vi "AutomatedTransfer_v2.vi"() -> ()   [LabVIEW 2013]
uses:
  controls/Control Configuration.ctl
  controls/Custom Controller Inputs.ctl
  controls/Controller Calcs.ctl
  controls/Observer Calcs.ctl
  controls/Other Calcs.ctl
  controls/UI Data.ctl
  controls/All FPGA Configuration Values.ctl
  controls/FPGA State.ctl
  controls/Raw Values.ctl
  Globals/Global - All UI Loop Stop.vi
  Globals/Global - UI Stream and Variable Connections.vi
  Globals/Global - Configuration Options.vi
  support/User Event - Stop/User Event - Stop.lvlib
  support/Message Queue/Message Queue.lvlib
  <vilib>/Analysis/NI_AALBase.lvlib
panel:
  in  "Switch to Safe State":bool
  in  "Exit":bool
  out "System Status":string="\n8/4/2014 6:26:47 PM: RT Error 91 - Variant To Data in RT Main.vi\n8/4/2014 6:26:32 PM: RT Error 91 - Variant To Data in RT Main.vi\n8/4/2014 6:26:21 PM: RT Error 91 - Variant To Data in RT Main.vi\n8/4/2014 6:26:03 PM: RT Error 91 - Variant To Data in RT Main.vi\n8/4/2014 6:25:47 PM: RT Error 91 - Variant To Data in RT Main.vi\n8/4/2014 6:25:36 PM: RT Error 91 - Variant To Data in RT Main.vi\n6/10/2014 3:19:43 PM: UI Error -1950679035 - Read Variable in AutomatedTransfer_v2.vi\n5/12/2014 3:31:58 PM: UI Error -314220 - Read Single Element from Stream in UI - Read Stream from RT.vi->UI Main.vi\n5/12/2014 3:31:58 PM: UI Error -314220 - Read Single Element from Stream in UI - Read Stream from RT.vi->UI Main.vi\n5/12/2014 3:31:58 PM: UI Error -314220 - Read Single Element from Stream in UI - Read Stream from RT.vi->UI Main.vi\n5/12/2014 3:31:58 PM: UI Error -314220 - Read Single Element from Stream in UI - Read Stream from RT.vi->UI Main.vi\n5/12/2014 3:31:58 PM: UI Error -314220 - Read Single Element from Stream in UI - Read Stream from RT.vi->UI Main.vi\n5/12/2014 3:31:58 PM: UI Error -314220 - Read Single Element from Stream in UI - Read Stream from RT.vi->UI Main.vi\n5/12/2014 3:31:58 PM: UI Error -314220 - Read Single Element from Stream in UI - Read Stream from RT.vi->UI Main.vi\n5/12/2014 3:31:58 PM: UI Error -314220 - Read Single Element from Stream in UI - Read Stream from RT.vi->UI Main.vi\n5/12/2014 3:31:58 PM: UI Error -314220 - Read Single Element from Stream in UI - Read Stream from RT.vi->UI Main.vi\n5/12/2014 3:31:58 PM: UI Error -314220 - Read Single Element from Stream in UI - Read Stream from RT.vi->UI Main.vi\n5/12/2014 3:31:58 PM: UI Error -314220 - Read Single Element from Stream in UI - Read Stream from RT.vi->UI Main.vi\n5/12/2014 3:31:58 PM: UI Error -314220 - Read Single Element from Stream in UI - Read Stream from RT.vi->UI Main.vi\n5/12/2014 3:31:58 PM: UI Error -314220 - Read Single Element from Stream in UI - Read Stream from RT.vi->UI Main.vi\n5/12/2014 3:31:58 PM: UI Error -314220 - Read Single Element from Stream in UI - Read Stream from RT.vi->UI Main.vi\n5/12/2014 3:31:58 PM: UI Error -314220 - Read Single Element from Stream in UI - Read Stream from RT.vi->UI Main.vi\n5/12/2014 3:31:58 PM: UI Error -314220 - Read Single Element from Stream in UI - Read Stream from RT.vi->UI Main.vi\n5/12/2014 3:31:58 PM: UI Error -314220 - Write Single Element to Stream in UI Main.vi\n5/12/2014 3:31:36 PM: UI Error -314004 - Create Network Stream Writer Endpoint in UI - Initiate Connection.vi->UI Main.vi\n5/6/2014 11:02:04 PM: UI Error -314220 - Write Single Element to Stream in UI Main.vi"
  out "Current FPGA Control Mode":u16(ring) items=["Safe State", "Manual", "Control (PID)"]
  in  "Settings Tab":T1(tab)
  out "Stage stop position (mm):":dbl=99.99983984375 format="%#.2g"
  out "Test LED":bool
  out "Roller LED":bool=TRUE
  in  "Test control":bool
  in  "Disable test control":bool
  in  "Stage speed (mm/s):":dbl=21.0 min=0.2 max=21.0
  out "Force results (N)":cluster{dbl[], dbl[]}(graph)
  in  "Save Results":bool
  in  "Stop Test":bool
  in  "Run Test":bool
  in  "Stop dwell time (s):":dbl=2.0 min=0.0
  in  "Start dwell time (s):":dbl=2.0 min=0.0
  in  "Travel distance (mm):":dbl=50.0 min=-150.0 max=150.0 step=0.1
  in  "Contact force (N):":fxp<+/-,20,7>=4.0
  out "Measured contact force (N):":dbl
  out "Stage position (mm):":dbl format="%#.2g"
  out "Fthresh (N):":fxp<+/-,16,8>=2.0 format="%.3g"
  in  "Home position (mm)":dbl=3.5
  in  "Stop roller":bool
  in  "Speed (mm/s):":dbl=2.0 min=0.2 max=5.0
  in  "Contact roller":bool
  in  "Disable roller control":bool
  in  "Roller control":bool
  in  "Home Roller":bool
  in  "Auto tare":bool=TRUE
  out "Position (mm):":dbl
  out "Force (N):":dbl
  out "Max speed (mm/s):":dbl=21.0
  out "Max position (mm):":dbl=151.49760546875
  in  "Position (mm):":dbl=85.0 min=0.0 max=150.0 step=0.1
  in  "Stage speed (mm/s):":dbl=21.0 min=0.2 max=21.0
  out "Stage position (mm):":dbl=99.9996015625 format="%#.2g"
  in  "Go stage":bool
  in  "Stop stage":bool
  in  "Home stage":bool
  out "path":path
  out "Other Calcs":T2
  out "Observer Calcs":T3
  out "Controller Calcs":T4
  in  "Control period (ticks)":u32=40000
  in  "Find tare offset":bool=TRUE
  in  "Channel 3 Setpoint":fxp<+/-,16,5>
  in  "Channel 2 Setpoint":fxp<+/-,16,5>
  in  "Channel 1 Setpoint":fxp<+/-,20,7>=24.0
  in  "Channel 0 Setpoint":fxp<+/-,20,7>=4.0
  in  "Update Control Configuration":bool
  in  "Control Configurations":T5[](array[typedef])=[{"PID Gains"={"proportional gain (Kc)"=55.0, "integral gain (Kc*Ts/Ti)"=0.0, "derivative gain (Kc*Td/Ts)"=0.0}, "Output Range"={"output high"=50.0, "output low"=-50.0}}, {"PID Gains"={"proportional gain (Kc)"=0.0, "integral gain (Kc*Ts/Ti)"=0.0, "derivative gain (Kc*Td/Ts)"=0.0}, "Output Range"={"output high"=10.0, "output low"=-10.0}}, {"PID Gains"={"proportional gain (Kc)"=0.0, "integral gain (Kc*Ts/Ti)"=0.0, "derivative gain (Kc*Td/Ts)"=0.0}, "Output Range"={"output high"=10.0, "output low"=-10.0}}, {"PID Gains"={"proportional gain (Kc)"=0.0, "integral gain (Kc*Ts/Ti)"=0.0, "derivative gain (Kc*Td/Ts)"=0.0}, "Output Range"={"output high"=10.0, "output low"=-10.0}}]
  in  "Run Control":bool
  in  "Stop Control":bool
  in  "Custom Controller Inputs":T6={"Other Controller Gains"={"kvc (N/m)"=1.0, "ymod (-)"=0.0, "Mar (kg)"=0.0, "bp (kg/s)"=0.0, "Foff (N)"=0.16796875, "Fthresh (N)"=2.0}}
  out "Offset (N)":fxp<+/-,16,8>=0.16796875
  in  "Channel 3 Manual Value":fxp<+/-,16,5>
  in  "Channel 2 Manual Value":fxp<+/-,16,5>
  in  "Channel 1 Manual Value":fxp<+/-,16,5>
  in  "Channel 0 Manual Value":fxp<+/-,16,5>
  in  "Run Manual":bool
  in  "Stop Manual":bool
  in  "Retain data":bool
  out "F std":dbl=0.005665196330386121 format="%#_4g"
  out "F avg":dbl=-0.0348828125 format="%#_4g"
  in  "Clear Button":bool
  in  "Pause Button":bool
  in  "Save As Button":bool
  in  "Display frequency (Hz)":dbl=100.0 min=1.0 step=1.0
  out "Inputs (mV or V)":cluster{dbl[], dbl[]}[](graph)
  in  "Number of points":i32=500 min=1 max=999999999
  out "Force (N)":cluster{dbl[], dbl[]}(graph)
  out "V*":cluster{dbl[], dbl[]}(graph)
  out "Roller position (mm)":cluster{dbl[], dbl[]}(graph)
  out "Control loop frequency (Hz)":u32=4294967295
  out "Stage position (mm)":cluster{dbl[], dbl[]}(graph)
  out "Actual Loop Period (ticks)":u32
  out "Largest Contiguous Memory (bytes)":dbl(graph)
  out "CPU Usage (%)":dbl(graph)
  out "Connected?":bool=TRUE
  in  "Connect to Controller":bool
  in  "Controller Address":string="169.254.66.100"
  # "LabVIEW FPGA Control on CompactRIO"
  # "Connection Settings"
  # "Roller panel"
  # "Stage panel"
  # "To do: \n-Update Monitoring Loop Rate by changing Display Rate \n  Note: with 1 ms rate, the program hangs\n-Put 'stage position' in variable references\n-Clean up noise in load cell when V* acts"
  # "Warning: Home cannot be stopped"
  # "Test panel"
  # "Force Command (N)"
  # "Position Command (mm)"
  # "Current Command (Testing)"
  # "Control period and setpoint changes are sent to the target automatically."
  # "Control Configuration changes are sent to the target when you click \"Update Control Configurations\"."
  # "Not used"
  # "Not used"
  # "Not used"
  # "F ="
  # "+/-"
  # "N"
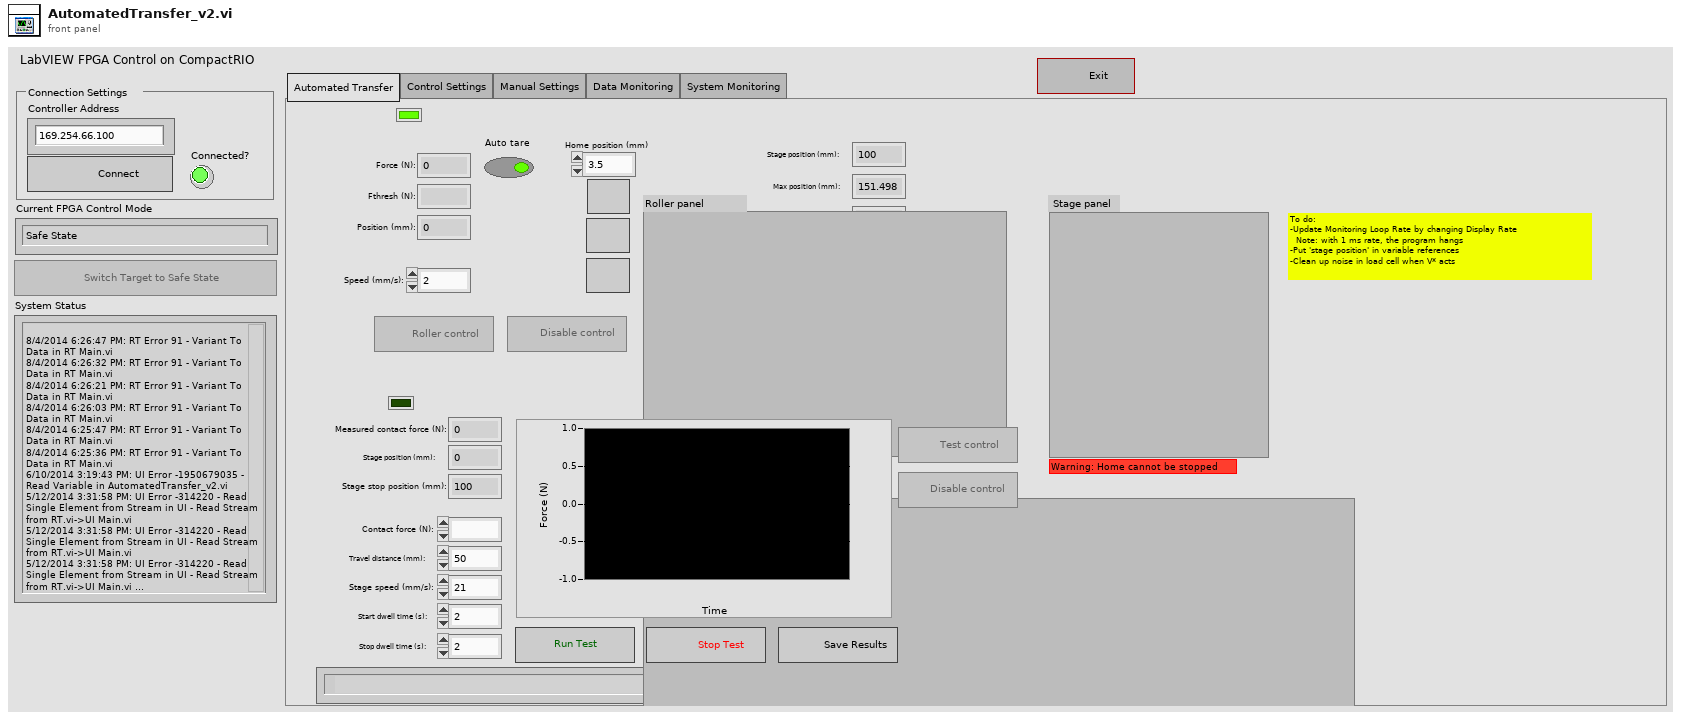
[diagram p1: front panel]
types:
  T1 = enum32{"Automated Transfer", "Control Settings", "Manual Settings", "Data Monitoring", "System Monitoring"}
  T2 = typedef "Other Calcs.ctl" = cluster{"k_1 (1/s)":fxp<+/-,20,7>, "k_2 (1/s)":fxp<+/-,20,7>, "Frr (N/s)":fxp<+/-,20,7>, "xrr (mm/s)":fxp<+/-,20,14>}
  T3 = typedef "Observer Calcs.ctl" = cluster{"bo (kg/s)":fxp<+/-,20,7>, "kso (N/m)":fxp<+/-,20,7>, "kiso (N/m)":fxp<+/-,20,7>}
  T4 = typedef "Controller Calcs.ctl" = cluster{"ba (kg/s)":fxp<+/-,20,7>, "ksa (N/m)":fxp<+/-,20,7>, "kisa (N/m)":fxp<+/-,20,7>, "k_backemf (Vs/m)":fxp<+/-,20,14>}
  T5 = typedef "Control Configuration.ctl" = cluster{"PID Gains":cluster{"proportional gain (Kc)":fxp<+/-,16,8>, "integral gain (Kc*Ts/Ti)":fxp<+/-,16,8>, "derivative gain (Kc*Td/Ts)":fxp<+/-,16,8>}, "Output Range":cluster{"output high":fxp<+/-,16,7>, "output low":fxp<+/-,16,7>}}
  T6 = typedef "Custom Controller Inputs.ctl" = cluster{"Other Controller Gains":cluster{"kvc (N/m)":fxp<+,16,12>, "ymod (-)":fxp<+/-,16,5>, "Mar (kg)":fxp<+/-,16,8>, "bp (kg/s)":fxp<+/-,16,5>, "Foff (N)":fxp<+/-,16,8>, "Fthresh (N)":fxp<+/-,16,5>}}
  T7 = typedef "UI Data.ctl" = cluster{"Switch to Safe State Ref":refnum<vi>, "Run Manual Ref":refnum<vi>, "Stop Manual Ref":refnum<vi>, "Run Control Ref":refnum<vi>, "Stop Control Ref":refnum<vi>, "Update Control Configurations Ref":refnum<vi>, "Ch 0 Setpoint Ref":refnum<vi>, "Ch 1 Setpoint Ref":refnum<vi>, "Ch 2 Setpoint Ref":refnum<vi>, "Ch 3 Setpoint Ref":refnum<vi>, "Ch 0 Manual Ref":refnum<vi>, "Ch 1 Manual Ref":refnum<vi>, "Ch 2 Manual Ref":refnum<vi>, "Ch 3 Manual Ref":refnum<vi>, "Control Configurations Ref":refnum<vi>, "Custom Controller Cluster Ref":refnum<vi>, "Control period (ticks) Ref":refnum<vi>, "Roller control":refnum<vi>, "Disable roller control":refnum<vi>, "Test control":refnum<vi>, "Disable test control":refnum<vi>, "Controller Calcs":refnum<vi>, "Observer Calcs":refnum<vi>, "Other Calcs":refnum<vi>}
  T8 = typedef "Message Queue.lvlib/All Message Queues.ctl" = cluster{"UI":refnum<queue>}
  T9 = enum16{"open", "replace", "create", "open or create", "replace or create", "replace or create with confirmation"}
  T10 = cluster{"Channel 0 Setpoint":fxp<+/-,20,7>, "Channel 1 Setpoint":fxp<+/-,20,7>, "Channel 2 Setpoint":fxp<+/-,16,5>, "Channel 3 Setpoint":fxp<+/-,16,5>}
  T11 = cluster{"Channel 0 Manual Value":fxp<+/-,16,5>, "Channel 1 Manual Value":fxp<+/-,16,5>, "Channel 2 Manual Value":fxp<+/-,16,5>, "Channel 3 Manual Value":fxp<+/-,16,5>}
  T12 = typedef "Variable References.ctl" = cluster{"CPU Usage":refnum<k21>, "Contiguous Memory":refnum<k21>, "Input Values":refnum<k21>, "Output Values":refnum<k21>, "FPGA Mode":refnum<k21>, "Actual Loop Period":refnum<k21>, "Controller Calcs":refnum<k21>, "Observer Calcs":refnum<k21>, "Other Calcs":refnum<k21>}
  T13 = typedef "Raw Values.ctl" = cluster{"Channel 0":fxp<+/-,20,7>, "Channel 1":fxp<+/-,20,7>, "Channel 2":fxp<+/-,20,7>, "Channel 3":fxp<+/-,20,14>}
  T14 = cluster{"Channel 0":dbl, "Channel 1":dbl, "Channel 2":dbl, "Channel 3":dbl}
  T15 = cluster{fxp<+/-,16,5>, "Channel 1 Manual Value":fxp<+/-,16,5>, "Channel 2 Manual Value":fxp<+/-,16,5>, "Channel 3 Manual Value":fxp<+/-,16,5>}
  T16 = cluster{"fixed-point type":fxp<+/-,16,5>, "Channel 1 Manual Value":fxp<+/-,16,5>, "Channel 2 Manual Value":fxp<+/-,16,5>, "Channel 3 Manual Value":fxp<+/-,16,5>}
  T17 = cluster{"Contact force (N): ":fxp<+/-,20,7>, "Channel 1 Setpoint":fxp<+/-,20,7>, "Channel 2 Setpoint":fxp<+/-,16,5>, "Channel 3 Setpoint":fxp<+/-,16,5>}
  T18 = cluster{"Message":string, "Message Data":variant}
  T19 = typedef "All FPGA Configuration Values.ctl" = cluster{"FPGA State":T20, "Manual Values":T13, "Setpoints":T13, "Control Configurations":T5[]}
  T20 = typedef "FPGA State.ctl" = enum16{"Safe State", "Manual", "Control (PID)"}
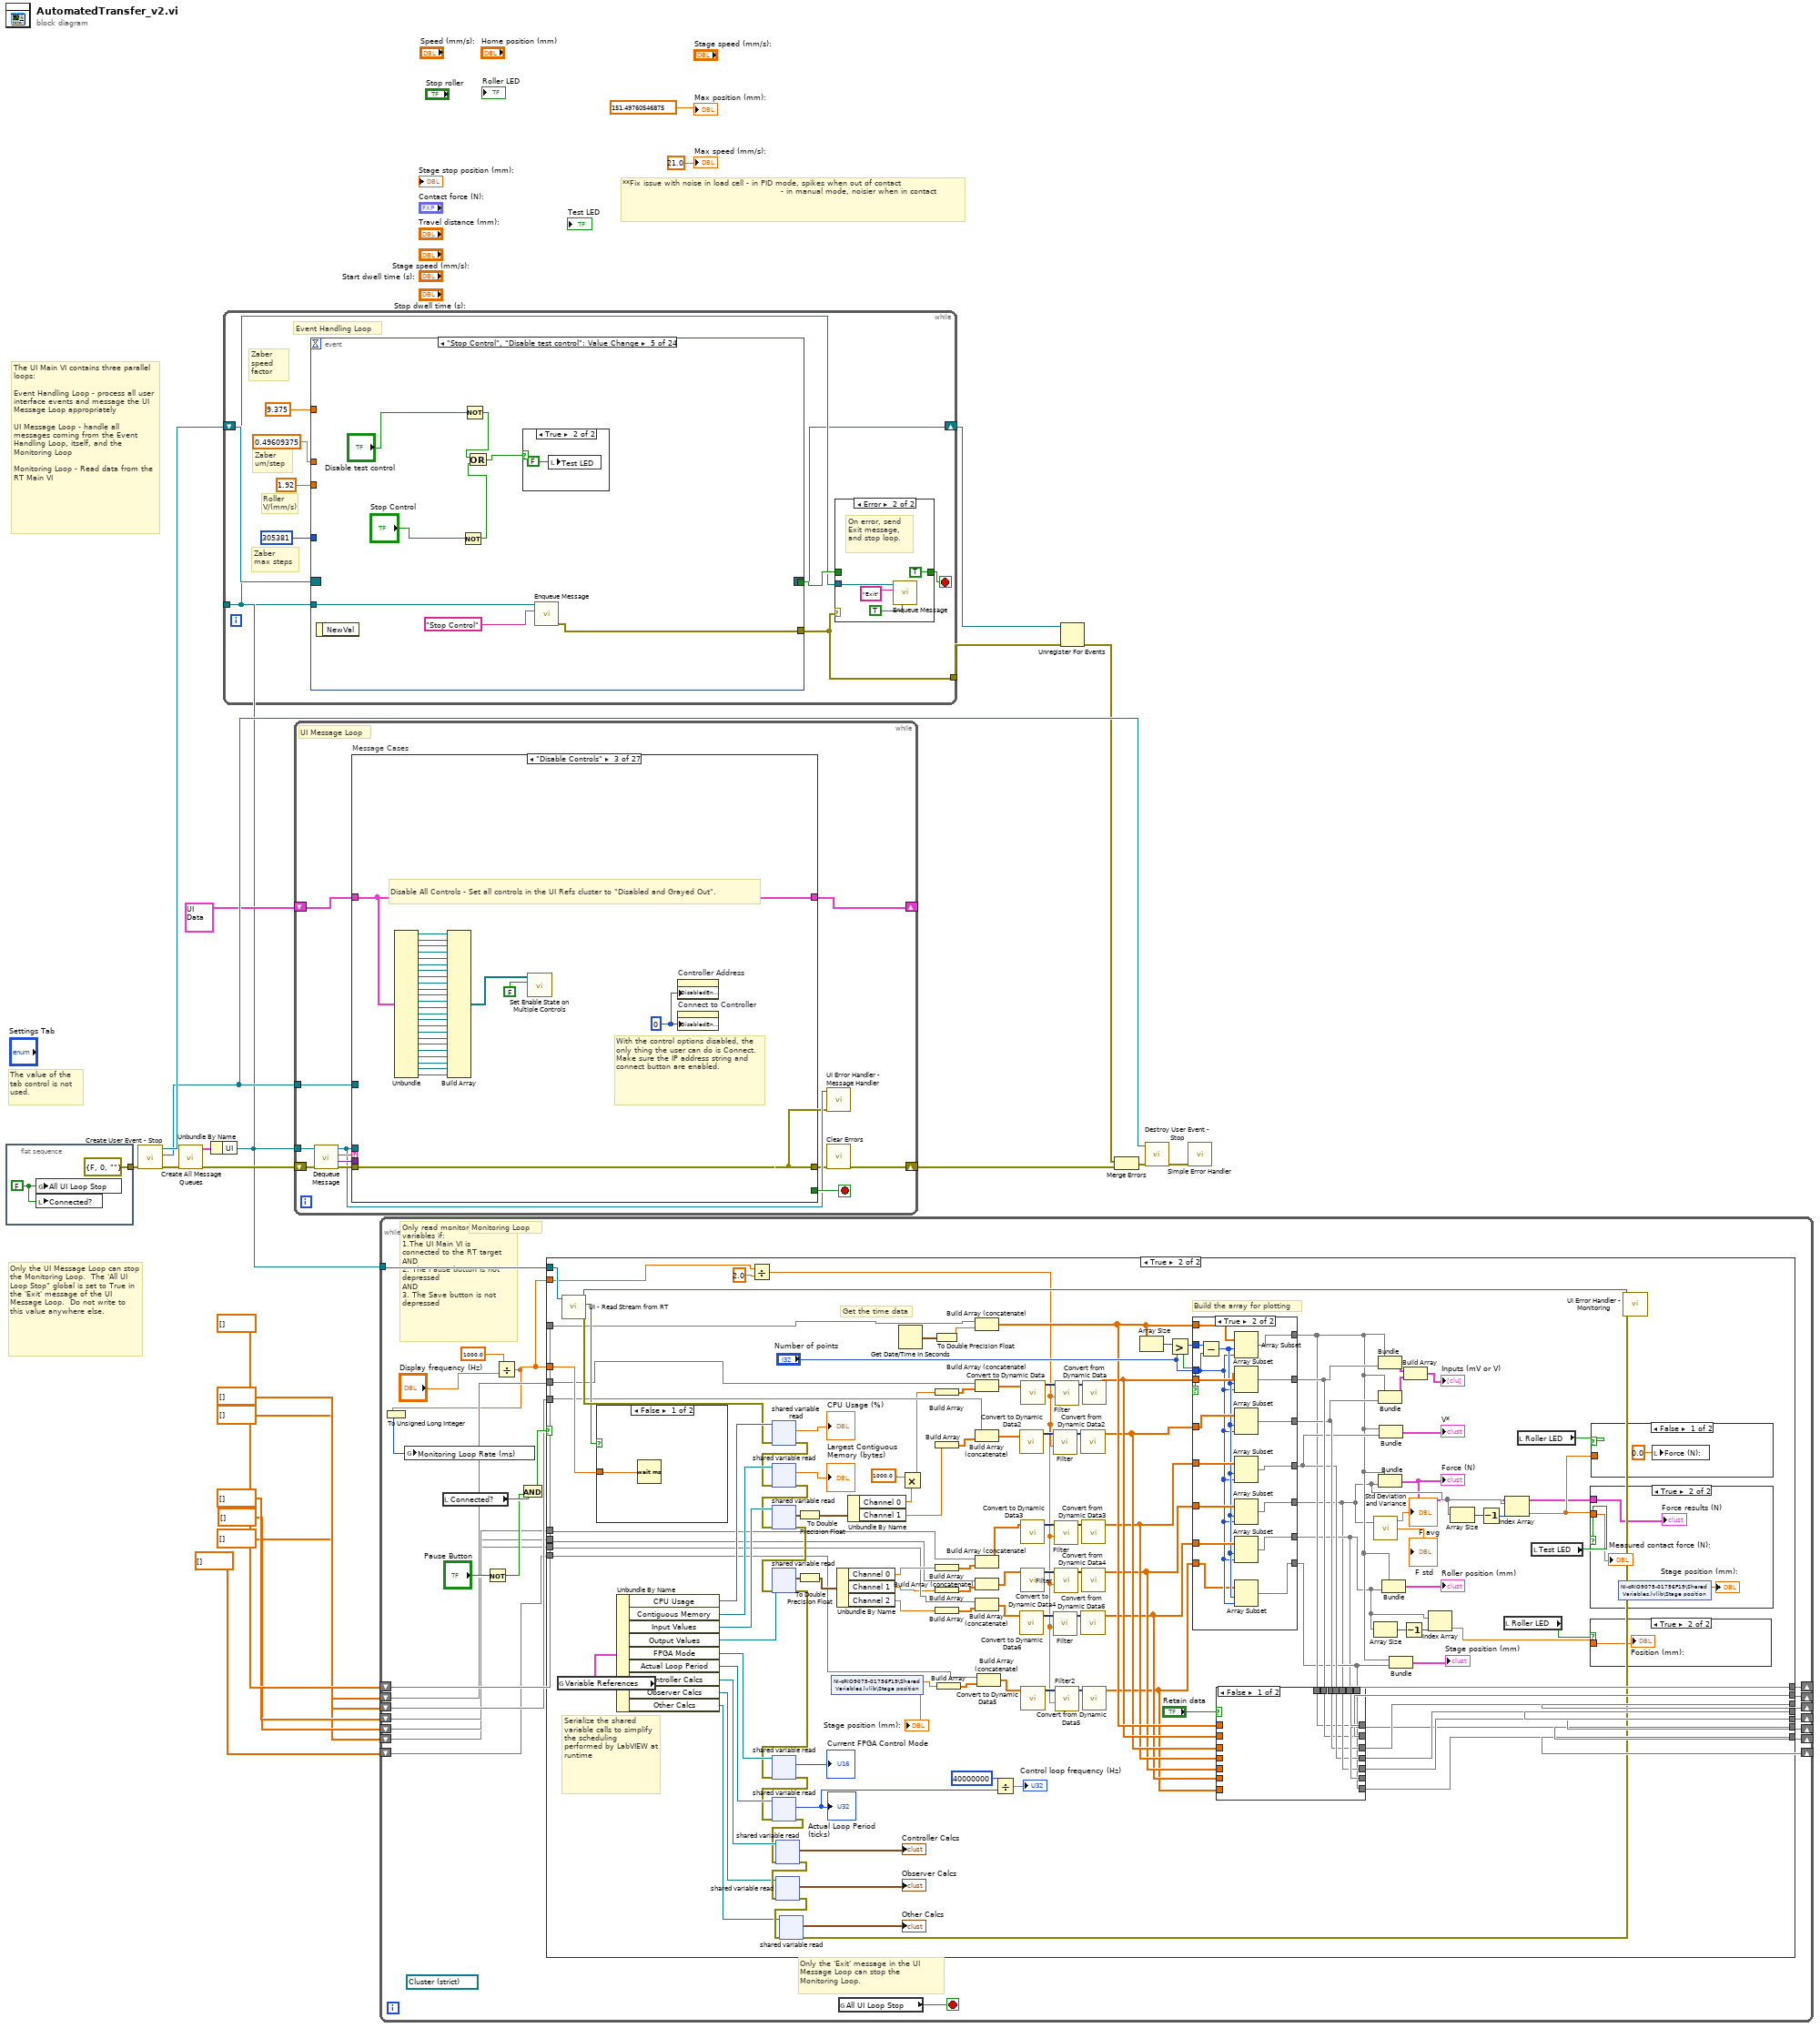
[diagram p0: block diagram]
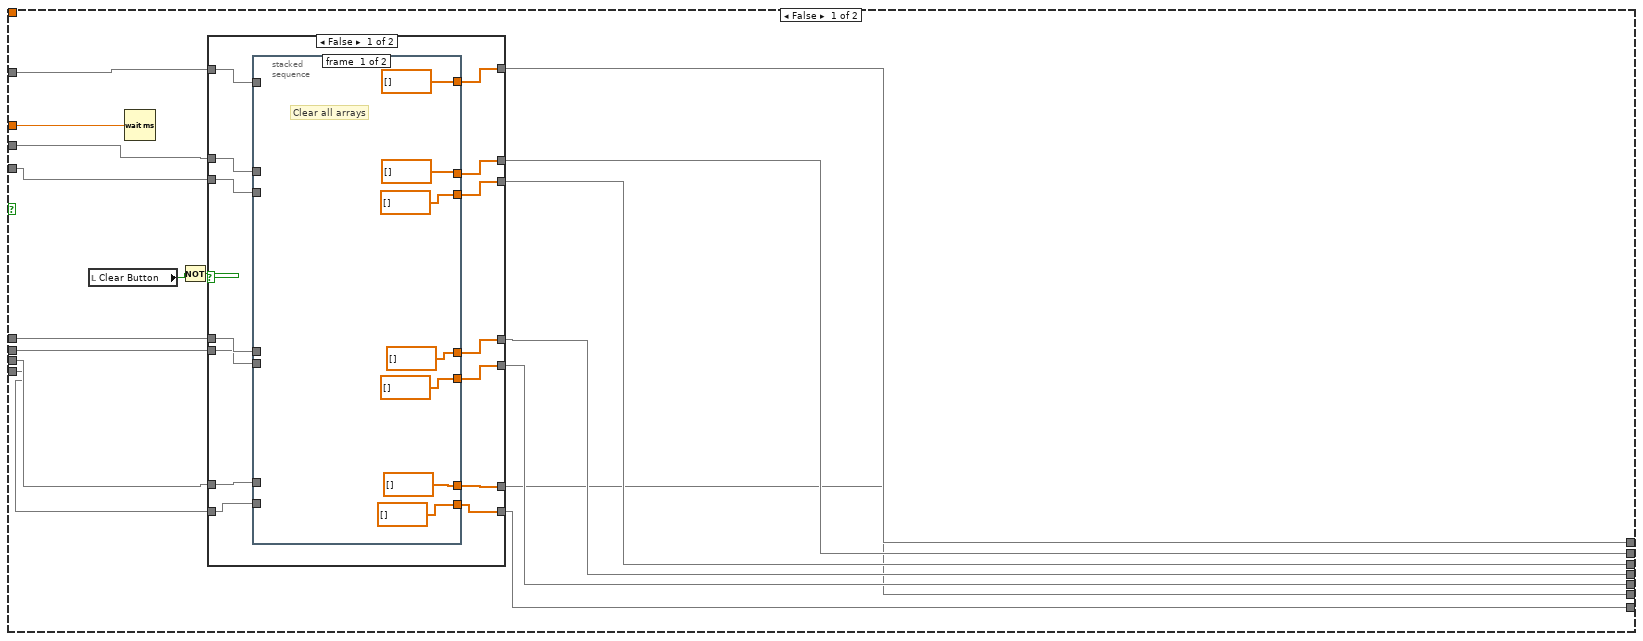
[diagram p2: hidden frame]
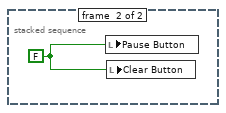
[diagram p3: hidden frame]
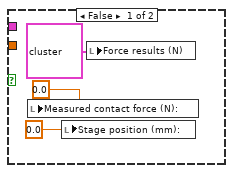
[diagram p5: hidden frame]
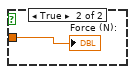
[diagram p6: hidden frame]
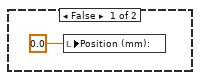
[diagram p7: hidden frame]
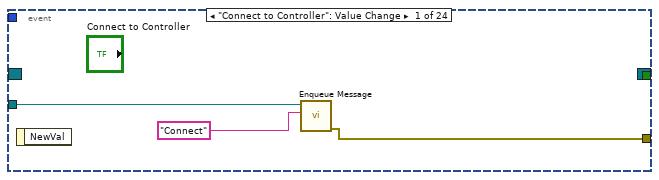
[diagram p12: hidden frame]
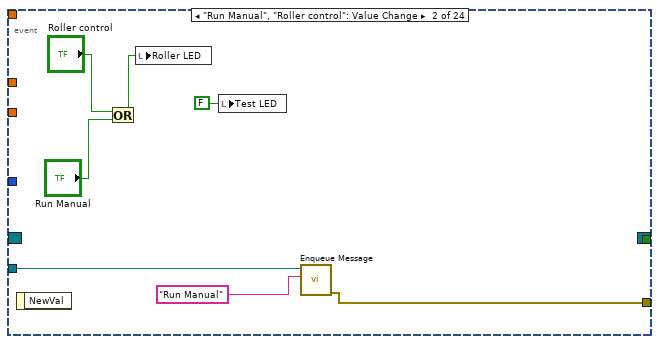
[diagram p13: hidden frame]
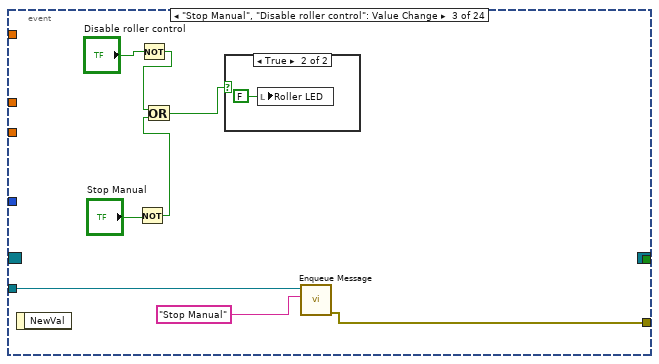
[diagram p14: hidden frame]
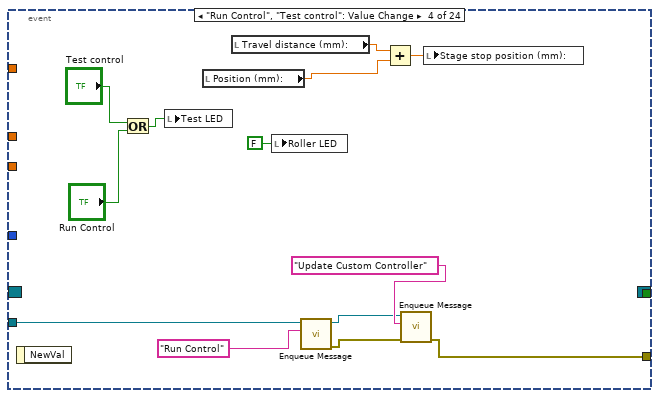
[diagram p16: hidden frame]
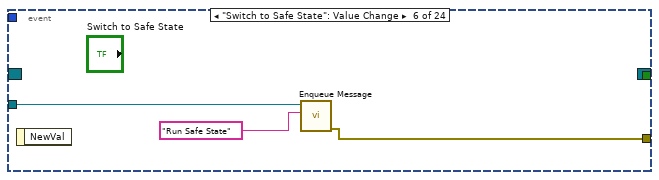
[diagram p18: hidden frame]
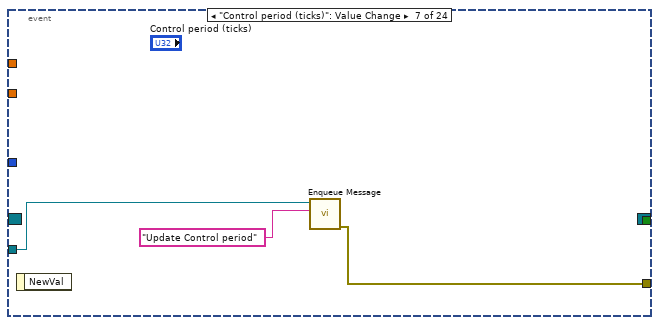
[diagram p19: hidden frame]
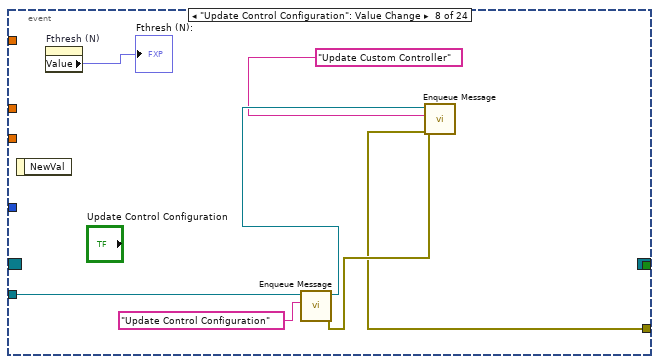
[diagram p20: hidden frame]
diagram:
  # "**Fix issue with noise in load cell - in PID mode, spikes when out of contact\n                                                          - in manual mode, noisier when in contact"
  # "The UI Main VI contains three parallel loops:\n\nEvent Handling Loop - process all user interface events and message the UI Message Loop appropriately\n\nUI Message Loop - handle all messages coming from the Event Handling Loop, itself, and the Monitoring Loop\n\nMonitoring Loop - Read data from the RT Main VI"
  # "The value of the tab control is not used."
  # "Only the UI Message Loop can stop the Monitoring Loop.  The 'All UI Loop Stop\" global is set to True in the 'Exit' message of the UI Message Loop.  Do not write to this value anywhere else."
  n1 = flat-sequence {
    tunnel: [errorcluster {"status"=FALSE, "code"=0, "source"=""} ("error in (no error)")] -> w10
    frame #0 {
      w24 = FALSE
      n2 = global write "Global - All UI Loop Stop.vi" "All UI Loop Stop"(w24) -> ()
      n3 = local write "Connected?"(w24) -> ()
    }
  }
  n4 = call "Create User Event - Stop.vi"("error in (no error)"=w10) -> ("error out"=w18:errorcluster, "User Event - Stop"=w19:refnum<user-event>, "Stop Event Registration Refnum"=w20:refnum<event-registration>)  [unwired: 8 in]
  n5 = call "Create All Message Queues.vi"("error in (no error)"=w18) -> ("error out"=w16:errorcluster, "Message Queues out"=w17:T8)  [unwired: 9 in]
  n6 = Unbundle By Name(w17) -> ("UI"=w11:refnum<queue>)
  n7 = while {
    tunnel: w11 -> [w31]
    tunnel: [w33] -> w22
    shift-right: [w30] -> w14
    shift-left: w20 -> [w32]
    stop <- w34 stop-if-true
    # "Zaber \nmax steps"
    # "Zaber \nspeed factor"
    # "Zaber \num/step"
    # "Roller \nV/(mm/s)"
    # "Event Handling Loop"
    n8 = event shown="[4] \"Stop Control\", \"Disable test control\": Value Change" {
      selector: w32 -> [_ _ _ _ _ _ _ _ _ _ _ _ _ _ _ _ _ _ _ _ _ _ _ _]
      dyn-events: [_ _ _ _ _ _ _ _ _ _ _ _ _ _ _ _ _ _ _ _ _ _ _ _] -> w30
      timeout: _ -> [_ _ _ _ _ _ _ _ _ _ _ _ _ _ _ _ _ _ _ _ _ _ _ _]
      tunnel: [_ _ _ _ _ _ _ _ _ _ _ _ _ _ _ _ _ _ _ _ _ TRUE ("Discard?") _ _] -> w35
      tunnel: w31 -> [w41 w48 w56 w71 w78 w82 w87 w94 w97 w106 w114 w139 w144 w175 w208 w219 w226 w270 w277 _ w296 _ _ _]
      tunnel: [w43 w50 w58 w67 w80 w84 w85 w90 w96 w105 w113 w142 w143 w174 w207 w220 w225 w269 w275 _ _ _ _ _] -> w33
      tunnel: 1.92 -> [_ _ _ _ _ _ _ _ _ _ _ _ _ w173 _ _ _ _ _ _ w295 _ _ _]
      tunnel: 0.49609375 -> [_ _ _ _ _ _ _ _ _ _ _ _ _ _ _ _ w224 _ _ _ w294 _ _ _]
      tunnel: 9.375 -> [_ _ _ _ _ _ _ _ _ _ _ _ _ _ _ _ w223 _ _ _ w293 _ _ _]
      tunnel: 305381 -> [_ _ _ _ _ _ _ _ _ _ _ _ _ _ _ _ w222 _ _ _ w292 _ _ _]
      event "Connect to Controller": Value Change {
        n9 = event-data() -> ()  [unwired: 1 in, 1 out]
        n10 = call "Enqueue Message.vi"("Message"="Connect", "Message Queue"=w41) -> ("error out"=w43:errorcluster)  [unwired: 8 in, 1 out]
      }
      event "Run Manual", "Roller control": Value Change {
        n11 = event-data() -> ()  [unwired: 1 in, 1 out]
        n12 = Or(x="Roller control", y="Run Manual") -> (x .or. y?=w45:bool)
        n13 = local write "Roller LED"(w45) -> ()
        n14 = local write "Test LED"(FALSE ("Test LED")) -> ()
        n15 = call "Enqueue Message.vi"("Message"="Run Manual", "Message Queue"=w48) -> ("error out"=w50:errorcluster)  [unwired: 8 in, 1 out]
      }
      event "Stop Manual", "Disable roller control": Value Change {
        n16 = event-data() -> ()  [unwired: 1 in, 1 out]
        n17 = Not(x="Stop Manual") -> (.not. x?=w53:bool)
        n18 = Not(x="Disable roller control") -> (.not. x?=w52:bool)
        n19 = Or(x=w52, y=w53) -> (x .or. y?=w51:bool)
        n20 = case shown="True" w51 {
          frame False {
          }
          frame True {
            n21 = local write "Roller LED"(FALSE) -> ()
          }
        }
        n22 = call "Enqueue Message.vi"("Message"="Stop Manual", "Message Queue"=w56) -> ("error out"=w58:errorcluster)  [unwired: 8 in, 1 out]
      }
      event "Run Control", "Test control": Value Change {
        n23 = event-data() -> ()  [unwired: 1 in, 1 out]
        n24 = Or(x="Test control", y="Run Control") -> (x .or. y?=w64:bool)
        n25 = local write "Test LED"(w64) -> ()
        n26 = local read "Position (mm):"() -> (w62:dbl)
        n27 = local read "Travel distance (mm):"() -> (w61:dbl)
        n28 = local write "Roller LED"(FALSE ("Roller LED")) -> ()
        n29 = call "Enqueue Message.vi"("Message"="Run Control", "Message Queue"=w71) -> ("error out"=w68:errorcluster, "dup Message Queue"=w69:refnum<queue>)  [unwired: 8 in]
        n30 = Add(x=w61, y=w62) -> (x+y=w60:dbl)
        n31 = call "Enqueue Message.vi"("error in (no error)"=w68, "Message"="Update Custom Controller", "Message Queue"=w69) -> ("error out"=w67:errorcluster)  [unwired: 7 in, 1 out]
        n32 = local write "Stage stop position (mm):"(w60) -> ()
      }
      event "Stop Control", "Disable test control": Value Change {
        n33 = event-data() -> ()  [unwired: 1 in, 1 out]
        n34 = Not(x="Stop Control") -> (.not. x?=w74:bool)
        n35 = Not(x="Disable test control") -> (.not. x?=w75:bool)
        n36 = Or(x=w75, y=w74) -> (x .or. y?=w73:bool)
        n37 = case shown="True" w73 {
          frame False {
          }
          frame True {
            n38 = local write "Test LED"(FALSE) -> ()
          }
        }
        n39 = call "Enqueue Message.vi"("Message"="Stop Control", "Message Queue"=w78) -> ("error out"=w80:errorcluster)  [unwired: 8 in, 1 out]
      }
      event "Switch to Safe State": Value Change {
        n40 = event-data() -> ()  [unwired: 1 in, 1 out]
        n41 = call "Enqueue Message.vi"("Message"="Run Safe State", "Message Queue"=w82) -> ("error out"=w84:errorcluster)  [unwired: 8 in, 1 out]
      }
      event "Control period (ticks)": Value Change {
        n42 = event-data() -> ()  [unwired: 1 in, 1 out]
        n43 = call "Enqueue Message.vi"("Message"="Update Control period", "Message Queue"=w87) -> ("error out"=w85:errorcluster)  [unwired: 8 in, 1 out]
      }
      event "Update Control Configuration": Value Change {
        n44 = event-data() -> ()  [unwired: 1 in, 1 out]
        n45 = property on="Fthresh (N)" class="DigNum (strict)"() -> ("Value"=→"Fthresh (N):":fxp<+/-,16,5>)  [unwired: 2 in, 2 out]
        n46 = call "Enqueue Message.vi"("Message"="Update Control Configuration", "Message Queue"=w94) -> ("error out"=w91:errorcluster, "dup Message Queue"=w92:refnum<queue>)  [unwired: 8 in]
        n47 = call "Enqueue Message.vi"("error in (no error)"=w91, "Message"="Update Custom Controller", "Message Queue"=w92) -> ("error out"=w90:errorcluster)  [unwired: 7 in, 1 out]
      }
      event "Channel 0 Setpoint", "Channel 1 Setpoint", "Channel 2 Setpoint", "Channel 3 Setpoint": Value Change {
        n48 = event-data() -> ()  [unwired: 1 in, 1 out]
        n49 = Bundle("Channel 0 Setpoint"="Channel 0 Setpoint", "Channel 1 Setpoint"="Channel 1 Setpoint", "Channel 2 Setpoint"="Channel 2 Setpoint", "Channel 3 Setpoint"="Channel 3 Setpoint") -> (w95:T10)  [unwired: 1 in]
        n50 = call "Enqueue Message.vi"("Message Data"=w95, "Message"="Update Setpoints", "Message Queue"=w97) -> ("error out"=w96:errorcluster)  [unwired: 7 in, 1 out]
      }
      event "Channel 0 Manual Value", "Channel 1 Manual Value", "Channel 2 Manual Value", "Channel 3 Manual Value": Value Change {
        n51 = event-data() -> ()  [unwired: 1 in, 1 out]
        n52 = Bundle("Channel 0 Manual Value"="Channel 0 Manual Value", "Channel 1 Manual Value"="Channel 1 Manual Value", "Channel 2 Manual Value"="Channel 2 Manual Value", "Channel 3 Manual Value"="Channel 3 Manual Value") -> (w103:T11)  [unwired: 1 in]
        n53 = call "Enqueue Message.vi"("Message Data"=w103, "Message"="Update Manual Values", "Message Queue"=w106) -> ("error out"=w105:errorcluster)  [unwired: 7 in, 1 out]
      }
      event "Find tare offset", "Auto tare": Value Change {
        # "When Auto tare is pressed, the offset force (N) is calculated. This value is automaticaly \ninputted into the Offset weight control of Other Controller Gains."
        n54 = event-data() -> ()  [unwired: 1 in, 1 out]
        n55 = property on="Foff (N)" class="DigNum (strict)"("Value"=fxp<+/-,16,8> 0.0) -> ()  [unwired: 2 in, 2 out]
        n56 = Or(x="Find tare offset", y="Auto tare") -> (x .or. y?=w115:bool)
        n57 = stacked-sequence {
          tunnel: 400 -> [w120 w133 _ _]
          tunnel: w115 -> [w119 _ _ _]
          tunnel: w114 -> [_ _ _ w137]
          tunnel: [_ _ _ w136] -> w113
          frame #0 {
            n58 = case shown="True" w119 {
              tunnel: w120 -> [_ w122]
              frame False {
                n59 = local write "Offset (N)"(0.0 ("Test")) -> ()
              }
              frame True {
                n60 = for {
                  N: w122 -> [_]
                  n61 = global read "Global - UI Stream and Variable Connections.vi" "Variable References"() -> (w126:T12)
                  n62 = Unbundle By Name(w126) -> ("Output Values"=w127:refnum<k21>)
                  n63 = shared-variable-read(w127) -> (w128:T13)  [unwired: 1 in, 3 out]
                  n64 = local read "Offset (N)"() -> (w125:fxp<+/-,16,8>)
                  n65 = To Double Precision Float(number=w128) -> (double precision float=w129:T14)
                  n66 = Unbundle(w129) -> ("Channel 1"=w123:dbl)  [unwired: 3 out]
                  n67 = Add(x=w123, y=w125) -> (x+y=w124:dbl)
                  n68 = local write "Offset (N)"(w124) -> ()
                  n69 = Wait (ms)(milliseconds to wait=u32 5) -> ()  [unwired: 1 out]
                }
              }
            }
          }
          frame #1 {
            n70 = local read "Offset (N)"() -> (w134:fxp<+/-,16,8>)
            n71 = To Double Precision Float(number=w133) -> (double precision float=w132:dbl)
            n72 = Divide(x=w134, y=w132) -> (x/y=w131:dbl)
            n73 = local write "Offset (N)"(w131) -> ()
          }
          frame #2 {
            n74 = local read "Offset (N)"() -> (w135:fxp<+/-,16,8>)
            n75 = property on="Foff (N)" class="DigNum (strict)"("Value"=w135) -> ()  [unwired: 2 in, 2 out]
          }
          frame #3 {
            n76 = call "Enqueue Message.vi"("Message"="Update Custom Controller", "Message Queue"=w137) -> ("error out"=w136:errorcluster)  [unwired: 8 in, 1 out]
          }
        }
        "Offset (N)" <- 0.0 ("Offset weight (N)")
      }
      event "Exit": Value Change {
        w140 = TRUE  # Priority Message
        # "The UI Message Loop handles sending the Exit message to other loops."
        n77 = event-data() -> ()  [unwired: 1 in, 1 out]
        n78 = call "Enqueue Message.vi"("Priority Message? (F)"=w140, "Message"="Exit", "Message Queue"=w139) -> ("error out"=w142:errorcluster)  [unwired: 7 in, 1 out]
      }
      event "Home Roller": Value Change {
        n79 = event-data() -> ()  [unwired: 1 in, 1 out]
        n80 = for {
          N: 3 -> [_]
          tunnel: w144 -> [w147]
          tunnel: [w146] -> w143
          i -> [w148]
          n81 = case shown="2" w148 {
            tunnel: w147 -> [_ w150 _ w170]
            tunnel: [_ w149 _ w169] -> w146
            frame Default {
            }
            frame 0 {
              # "V/(mm/s)"
              n82 = local read "Speed (mm/s):"() -> (w152:dbl)
              n83 = local read "Channel 1 Manual Value"() -> (w157:fxp<+/-,16,5>)
              n84 = local read "Channel 2 Manual Value"() -> (w156:fxp<+/-,16,5>)
              n85 = local read "Channel 3 Manual Value"() -> (w155:fxp<+/-,16,5>)
              n86 = Multiply(x=w152, y=-1.92) -> (x*y=w154:dbl)
              n87 = To Fixed-Point(number=w154) -> (fixed-point=w151:fxp<+/-,16,5>)  [unwired: 1 in]
              n88 = local write "Channel 0 Manual Value"(w151) -> ()
              n89 = Bundle(w151, "Channel 1 Manual Value"=w157, "Channel 2 Manual Value"=w156, "Channel 3 Manual Value"=w155) -> (w158:T15)  [unwired: 1 in]
              n90 = call "Enqueue Message.vi"("Message Data"=w158, "Message"="Home roller", "Message Queue"=w150) -> ("error out"=w149:errorcluster)  [unwired: 7 in, 1 out]
            }
            frame 1 {
              n91 = while {
                stop <- w163 stop-if-true
                n92 = local read "Home position (mm)"() -> (w160:dbl)
                n93 = local read "Position (mm):"() -> (w161:dbl)
                n94 = local read "Stop roller"() -> (w162:bool)
                n95 = Less?(x=w161, y=w160) -> (x < y?=w164:bool)
                n96 = Or(x=w164, y=w162) -> (x .or. y?=w163:bool)
              }
            }
            frame 2 {
              w168 = fxp<+/-,16,5> 0.0 ("fixed-point type")
              n97 = local read "Channel 3 Manual Value"() -> (w165:fxp<+/-,16,5>)
              n98 = local read "Channel 2 Manual Value"() -> (w166:fxp<+/-,16,5>)
              n99 = local read "Channel 1 Manual Value"() -> (w167:fxp<+/-,16,5>)
              n100 = local write "Channel 0 Manual Value"(w168) -> ()
              n101 = Bundle("fixed-point type"=w168, "Channel 1 Manual Value"=w167, "Channel 2 Manual Value"=w166, "Channel 3 Manual Value"=w165) -> (w171:T16)  [unwired: 1 in]
              n102 = call "Enqueue Message.vi"("Message Data"=w171, "Message"="Contact roller", "Message Queue"=w170) -> ("error out"=w169:errorcluster)  [unwired: 7 in, 1 out]
            }
          }
        }
      }
      event "Contact roller": Value Change {
        n103 = event-data() -> ()  [unwired: 1 in, 1 out]
        n104 = for {
          N: 3 -> [_]
          tunnel: w175 -> [w179]
          tunnel: [w178] -> w174
          tunnel: w173 -> [w177]
          i -> [w180]
          n105 = case shown="1" w180 {
            tunnel: w179 -> [_ w183 _ w199]
            tunnel: [_ w182 _ w198] -> w178
            tunnel: w177 -> [_ w181 _ _]
            frame Default {
            }
            frame 0 {
              n106 = local read "Speed (mm/s):"() -> (w188:dbl)
              n107 = local read "Channel 3 Manual Value"() -> (w184:fxp<+/-,16,5>)
              n108 = local read "Channel 1 Manual Value"() -> (w186:fxp<+/-,16,5>)
              n109 = local read "Channel 2 Manual Value"() -> (w185:fxp<+/-,16,5>)
              n110 = Multiply(x=w188, y=w181) -> (x*y=w189:dbl)
              n111 = To Fixed-Point(number=w189) -> (fixed-point=w187:fxp<+/-,16,5>)  [unwired: 1 in]
              n112 = local write "Channel 0 Manual Value"(w187) -> ()
              n113 = Bundle(w187, "Channel 1 Manual Value"=w186, "Channel 2 Manual Value"=w185, "Channel 3 Manual Value"=w184) -> (w190:T15)  [unwired: 1 in]
              n114 = call "Enqueue Message.vi"("Message Data"=w190, "Message"="Contact roller", "Message Queue"=w183) -> ("error out"=w182:errorcluster)  [unwired: 7 in, 1 out]
            }
            frame 1 {
              n115 = while {
                stop <- w194 stop-if-true
                n116 = local read "Fthresh (N):"() -> (w192:fxp<+/-,16,8>)
                n117 = local read "Force (N):"() -> (w197:dbl)
                n118 = local read "Stop roller"() -> (w195:bool)
                n119 = To Double Precision Float(number=w192) -> (double precision float=w193:dbl)
                n120 = Greater?(x=w197, y=w193) -> (0:w196:bool)
                n121 = Or(x=w196, y=w195) -> (x .or. y?=w194:bool)
              }
            }
            frame 2 {
              w200 = fxp<+/-,16,5> 0.0 ("fixed-point type")
              n122 = local read "Channel 1 Manual Value"() -> (w203:fxp<+/-,16,5>)
              n123 = local read "Channel 2 Manual Value"() -> (w202:fxp<+/-,16,5>)
              n124 = local read "Channel 3 Manual Value"() -> (w201:fxp<+/-,16,5>)
              n125 = local write "Channel 0 Manual Value"(w200) -> ()
              n126 = Bundle("fixed-point type"=w200, "Channel 1 Manual Value"=w203, "Channel 2 Manual Value"=w202, "Channel 3 Manual Value"=w201) -> (w204:T16)  [unwired: 1 in]
              n127 = call "Enqueue Message.vi"("Message Data"=w204, "Message"="Contact roller", "Message Queue"=w199) -> ("error out"=w198:errorcluster)  [unwired: 7 in, 1 out]
            }
          }
        }
      }
      event "Stop roller": Value Change {
        n128 = event-data() -> ()  [unwired: 1 in, 1 out]
        n129 = local read "Channel 2 Manual Value"() -> (w210:fxp<+/-,16,5>)
        n130 = local read "Channel 1 Manual Value"() -> (w211:fxp<+/-,16,5>)
        n131 = local read "Channel 3 Manual Value"() -> (w209:fxp<+/-,16,5>)
        n132 = Bundle("fixed-point type"=fxp<+/-,16,5> 0.0, "Channel 1 Manual Value"=w211, "Channel 2 Manual Value"=w210, "Channel 3 Manual Value"=w209) -> (w213:T16)  [unwired: 1 in]
        n133 = call "Enqueue Message.vi"("Message Data"=w213, "Message"="Stop roller", "Message Queue"=w208) -> ("error out"=w207:errorcluster)  [unwired: 7 in, 1 out]
      }
      event "Home stage": Value Change {
        n134 = event-data() -> ()  [unwired: 1 in, 1 out]
        n135 = Bundle(1, 1, 0, 1) -> (w214:cluster{i32, i32, i32, i32})  [unwired: 1 in]
        n136 = call "Enqueue Message.vi"("Message Data"=w214, "Message"="Home stage", "Message Queue"=w219) -> ("error out"=w220:errorcluster)  [unwired: 7 in, 1 out]
      }
      event "Go stage": Value Change {
        n137 = event-data() -> ()  [unwired: 1 in, 1 out]
        n138 = for {
          N: 2 -> [_]
          tunnel: w226 -> [w232]
          tunnel: [w231] -> w225
          tunnel: w224 -> [w230]
          tunnel: w223 -> [w229]
          tunnel: w222 -> [w228]
          i -> [w233]
          n139 = case shown="1" w233 {
            tunnel: w232 -> [_ w248 w261]
            tunnel: [_ w247 w260] -> w231
            tunnel: w230 -> [_ w235 _]
            tunnel: w229 -> [_ w234 _]
            tunnel: w228 -> [_ _ w251]
            frame Default {
            }
            frame 0 {
              n140 = local read "Stage speed (mm/s):"() -> (w241:dbl)
              n141 = Multiply(x=w234, y=w235) -> (x*y=w245:dbl)
              n142 = Divide(x=w245, y=1000.0) -> (x/y=w246:dbl)
              n143 = Divide(x=1.0, y=w246) -> (x/y=w242:dbl)
              n144 = Multiply(x=w241, y=w242) -> (x*y=w240:dbl)
              n145 = To Long Integer(number=w240) -> (32bit integer=w239:i32)
              n146 = Bundle(1, 42, w239, 1) -> (w249:cluster{i32, i32, i32, i32})  [unwired: 1 in]
              n147 = call "Enqueue Message.vi"("Message Data"=w249, "Message"="Update stage speed", "Message Queue"=w248) -> ("error out"=w247:errorcluster)  [unwired: 7 in, 1 out]
            }
            frame 1 {
              n148 = local read "Max position (mm):"() -> (w257:dbl)
              n149 = Divide(x=w251, y=w257) -> (x/y=w258:dbl)
              n150 = Multiply(x="Position (mm):", y=w258) -> (x*y=w259:dbl)
              n151 = To Long Integer(number=w259) -> (32bit integer=w252:i32)
              n152 = Bundle(1, 20, w252, 1) -> (w262:cluster{i32, i32, i32, i32})  [unwired: 1 in]
              n153 = call "Enqueue Message.vi"("Message Data"=w262, "Message"="Go stage", "Message Queue"=w261) -> ("error out"=w260:errorcluster)  [unwired: 7 in, 1 out]
            }
          }
        }
      }
      event "Stop stage", "Stop Test": Value Change {
        n154 = event-data() -> ()  [unwired: 1 in, 1 out]
        n155 = case shown="False" "Stop Test" {
          frame False {
            n156 = local write "Pause Button"(FALSE ("Pause Button")) -> ()
          }
          frame True {
          }
        }
        n157 = Bundle(1, 23, 0, 1) -> (w271:cluster{i32, i32, i32, i32})  [unwired: 1 in]
        n158 = call "Enqueue Message.vi"("Message Data"=w271, "Message"="Stop stage", "Message Queue"=w270) -> ("error out"=w269:errorcluster)  [unwired: 7 in, 1 out]
      }
      event "Contact force (N):": Value Change {
        n159 = event-data() -> ()  [unwired: 1 in, 1 out]
        n160 = local read "Contact force (N):"() -> (w274:fxp<+/-,20,7>)
        n161 = local read "Channel 2 Setpoint"() -> (w279:fxp<+/-,16,5>)
        n162 = local read "Channel 3 Setpoint"() -> (w280:fxp<+/-,16,5>)
        n163 = local read "Channel 1 Setpoint"() -> (w278:fxp<+/-,20,7>)
        n164 = Bundle("Contact force (N):"=w274, "Channel 1 Setpoint"=w278, "Channel 2 Setpoint"=w279, "Channel 3 Setpoint"=w280) -> (w281:T17)  [unwired: 1 in]
        n165 = call "Enqueue Message.vi"("Message Data"=w281, "Message"="Update Setpoints", "Message Queue"=w277) -> ("error out"=w275:errorcluster)  [unwired: 7 in, 1 out]
        n166 = local write "Channel 0 Setpoint"(w274) -> ()
      }
      event "Travel distance (mm):": Value Change {
        # "Keep the inputted travel distance consistent with the range 0-->150 mm"
        n167 = event-data() -> ()  [unwired: 1 in, 1 out]
        n168 = local read "Travel distance (mm):"() -> (w288:dbl)
        n169 = local read "Stage position (mm):"() -> (w289:dbl)
        n170 = Add(x=w289, y=w288) -> (x+y=w282:dbl)
        n171 = Greater?(x=w282, y=0.0) -> (0:w284:bool)
        n172 = Greater Or Equal?(x=150.0, y=w282) -> (x >= y?=w285:bool)
        n173 = And(x=w285, y=w284) -> (x .and. y?=w283:bool)
        n174 = case shown="False" w283 {
          tunnel: w282 -> [w290 w291]
          frame False {
            n175 = local write "Stage stop position (mm):"(w290) -> ()
            n176 = call "Display Message to User"() -> ()  [unwired: 10 in, 2 out]
          }
          frame True {
            n177 = local write "Stage stop position (mm):"(w291) -> ()
          }
        }
      }
      event "Run Test": Value Change {
        n178 = event-data() -> ()  [unwired: 1 in, 1 out]
        n179 = for {
          N: 11 -> [_]
          tunnel: w296 -> [w303]
          tunnel: [w302] -> _
          tunnel: w295 -> [w301]
          tunnel: w294 -> [w300]
          tunnel: w293 -> [w299]
          tunnel: w292 -> [w298]
          i -> [w304]
          n180 = case shown="2" w304 {
            tunnel: w303 -> [_ _ w309 w328 _ _ w344 _ _ _ _ _]
            tunnel: [_ _ w310 w327 _ _ w343 _ _ _ _ _] -> w302
            tunnel: w301 -> [_ _ _ _ _ _ _ _ _ _ _ _]
            tunnel: w300 -> [_ _ w307 _ _ _ _ _ _ _ _ _]
            tunnel: w299 -> [_ _ w308 _ _ _ _ _ _ _ _ _]
            tunnel: w298 -> [_ _ _ _ _ _ w341 _ _ _ _ _]
            frame Default {
            }
            frame 0 {
              w305 = 2
              n181 = property on="Stage speed (mm/s):" class="DigNum (strict)"("DisabledEnum"=w305) -> ()  [unwired: 2 in, 2 out]
              n182 = property on="Position (mm):" class="DigNum (strict)"("DisabledEnum"=w305) -> ()  [unwired: 2 in, 2 out]
              n183 = property on="Contact force (N):" class="DigNum (strict)"("DisabledEnum"=w305) -> ()  [unwired: 2 in, 2 out]
              n184 = property on="Travel distance (mm):" class="DigNum (strict)"("DisabledEnum"=w305) -> ()  [unwired: 2 in, 2 out]
              n185 = property on="Stage speed (mm/s):" class="DigNum (strict)"("DisabledEnum"=w305) -> ()  [unwired: 2 in, 2 out]
              n186 = property on="Start dwell time (s):" class="DigNum (strict)"("DisabledEnum"=w305) -> ()  [unwired: 2 in, 2 out]
              n187 = property on="Stop dwell time (s):" class="DigNum (strict)"("DisabledEnum"=w305) -> ()  [unwired: 2 in, 2 out]
            }
            frame 1 {
              n188 = local read "Stage speed (mm/s):"() -> (w306:dbl)
              n189 = Multiply(x=w308, y=w307) -> (x*y=w314:dbl)
              n190 = Divide(x=w314, y=1000.0) -> (x/y=w313:dbl)
              n191 = Divide(x=1.0, y=w313) -> (x/y=w317:dbl)
              n192 = Multiply(x=w306, y=w317) -> (x*y=w318:dbl)
              n193 = To Long Integer(number=w318) -> (32bit integer=w319:i32)
              n194 = Bundle(1, 42, w319, 1) -> (w312:cluster{i32, i32, i32, i32})  [unwired: 1 in]
              n195 = call "Enqueue Message.vi"("Message Data"=w312, "Message"="Update stage speed", "Message Queue"=w309) -> ("error out"=w310:errorcluster)  [unwired: 7 in, 1 out]
            }
            frame 2 {
              n196 = local read "Channel 3 Setpoint"() -> (w326:fxp<+/-,16,5>)
              n197 = local read "Channel 2 Setpoint"() -> (w325:fxp<+/-,16,5>)
              n198 = local read "Contact force (N):"() -> (w323:fxp<+/-,20,7>)
              n199 = local read "Channel 1 Setpoint"() -> (w324:fxp<+/-,20,7>)
              n200 = Bundle("Contact force (N):"=w323, "Channel 1 Setpoint"=w324, "Channel 2 Setpoint"=w325, "Channel 3 Setpoint"=w326) -> (w329:T17)  [unwired: 1 in]
              n201 = local write "Channel 0 Setpoint"(w323) -> ()
              n202 = call "Enqueue Message.vi"("Message Data"=w329, "Message"="Update Setpoints", "Message Queue"=w328) -> ("error out"=w327:errorcluster)  [unwired: 7 in, 1 out]
            }
            frame 3 {
              n203 = flat-sequence {
                frame #0 {
                  n204 = local write "Number of points"(99999999 ("Number of points")) -> ()
                }
                frame #1 {
                  n205 = local write "Pause Button"(TRUE) -> ()
                  n206 = local write "Clear Button"(TRUE) -> ()
                }
              }
            }
            frame 4 {
              n207 = local read "Start dwell time (s):"() -> (w336:dbl)
              n208 = Multiply(x=w336, y=1000.0) -> (x*y=w335:dbl)
              n209 = Wait (ms)(milliseconds to wait=w335) -> ()  [unwired: 1 out]
            }
            frame 5 {
              n210 = local read "Stage position (mm):"() -> (w337:dbl)
              n211 = local read "Travel distance (mm):"() -> (w339:dbl)
              n212 = local read "Max position (mm):"() -> (w340:dbl)
              n213 = Divide(x=w341, y=w340) -> (x/y=w349:dbl)
              n214 = Add(x=w339, y=w337) -> (x+y=w338:dbl)
              n215 = Multiply(x=w338, y=w349) -> (x*y=w350:dbl)
              n216 = To Long Integer(number=w350) -> (32bit integer=w345:i32)
              n217 = Bundle(1, 20, w345, 1) -> (w342:cluster{i32, i32, i32, i32})  [unwired: 1 in]
              n218 = call "Enqueue Message.vi"("Message Data"=w342, "Message"="Go stage", "Message Queue"=w344) -> ("error out"=w343:errorcluster)  [unwired: 7 in, 1 out]
            }
            frame 6 {
              n219 = while {
                stop <- w369 stop-if-true
                w357 = 100.0 ("y")
                w356 = 100.0 ("x")
                n220 = local read "Stage stop position (mm):"() -> (w361:dbl)
                n221 = shared-variable "NI-cRIO9075-01756F19\\Shared Variables.lvlib\\Stage position"() -> (w358:dbl)  [unwired: 1 in, 1 out]
                n222 = local read "Stop Test"() -> (w365:bool)
                n223 = local read "Test LED"() -> (w367:bool)
                n224 = Multiply(x=w358, y=w356) -> (x*y=w363:dbl)
                n225 = Multiply(x=w361, y=w357) -> (x*y=w362:dbl)
                n226 = Not(x=w367) -> (.not. x?=w364:bool)
                n227 = To Long Integer(number=w363) -> (32bit integer=w360:i32)
                n228 = To Long Integer(number=w362) -> (32bit integer=w355:i32)
                n229 = Divide(x=w355, y=w357) -> (x/y=w354:dbl)
                n230 = Divide(x=w360, y=w356) -> (x/y=w359:dbl)
                n231 = Or(x=w365, y=w364) -> (x .or. y?=w366:bool)
                n232 = To Long Integer(number=w354) -> (32bit integer=w352:i32)
                n233 = To Long Integer(number=w359) -> (32bit integer=w353:i32)
                n234 = Equal?(x=w353, y=w352) -> (x = y?=w368:bool)
                n235 = Or(x=w368, y=w366) -> (x .or. y?=w369:bool)
              }
            }
            frame 7 {
              n236 = local read "Stop Test"() -> (w370:bool)
              n237 = case shown="True" w370 {
                frame False {
                }
                frame True {
                  n238 = local write "Stop dwell time (s):"(0.0 ("Stop dwell time (s):")) -> ()
                }
              }
            }
            frame 8 {
              n239 = local read "Stop dwell time (s):"() -> (w372:dbl)
              n240 = Multiply(x=w372, y=1000.0) -> (x*y=w374:dbl)
              n241 = Wait (ms)(milliseconds to wait=w374) -> ()  [unwired: 1 out]
            }
            frame 9 {
              n242 = local write "Stop Test"(TRUE) -> ()
              n243 = local write "Pause Button"(TRUE) -> ()
            }
            frame 10 {
              w379 = 0
              n244 = local write "Number of points"(500 ("Number of points")) -> ()
              n245 = local write "Travel distance (mm):"(0.0 ("Travel distance (mm):")) -> ()
              n246 = property on="Stage speed (mm/s):" class="DigNum (strict)"("DisabledEnum"=w379) -> ()  [unwired: 2 in, 2 out]
              n247 = property on="Position (mm):" class="DigNum (strict)"("DisabledEnum"=w379) -> ()  [unwired: 2 in, 2 out]
              n248 = property on="Contact force (N):" class="DigNum (strict)"("DisabledEnum"=w379) -> ()  [unwired: 2 in, 2 out]
              n249 = property on="Travel distance (mm):" class="DigNum (strict)"("DisabledEnum"=w379) -> ()  [unwired: 2 in, 2 out]
              n250 = property on="Stage speed (mm/s):" class="DigNum (strict)"("DisabledEnum"=w379) -> ()  [unwired: 2 in, 2 out]
              n251 = property on="Start dwell time (s):" class="DigNum (strict)"("DisabledEnum"=w379) -> ()  [unwired: 2 in, 2 out]
              n252 = property on="Stop dwell time (s):" class="DigNum (strict)"("DisabledEnum"=w379) -> ()  [unwired: 2 in, 2 out]
            }
          }
        }
      }
      event User Event {
        # "The Message Handling Loop processed an \"Exit\" message, which fired this event to stop the Event Handling Loop."
        n253 = event-data() -> ()  [unwired: 1 in, 1 out]
      }
      event "Save As Button", "Save Results": Value Change {
        # "When Save As is pressed, V*, Force, and Position are saved."
        n254 = event-data() -> ()  [unwired: 1 in, 1 out]
        n255 = stacked-sequence {
          frame #0 {
            n256 = call "File Dialog"() -> ("selected path"=w383:path)  [unwired: 12 in, 3 out]
            n257 = local read "Stage position (mm)"() -> (w392:cluster{dbl[], dbl[]})
            n258 = local read "Roller position (mm)"() -> (w391:cluster{dbl[], dbl[]})
            n259 = local read "Force (N)"() -> (w389:cluster{dbl[], dbl[]})
            n260 = local read "V*"() -> (w390:cluster{dbl[], dbl[]})
            n261 = Unbundle(w392) -> (w408:dbl[], w409:dbl[])
            n262 = Unbundle(w389) -> (w394:dbl[])  [unwired: 1 out]
            n263 = Unbundle(w391) -> (w393:dbl[])  [unwired: 1 out]
            n264 = Unbundle(w390) -> (w396:dbl[])  [unwired: 1 out]
            n265 = Array Max & Min(array=w408) -> (min value=w406:dbl)  [unwired: 3 out]
            n266 = Subtract(x=w408, y=w406) -> (x-y=w407:dbl[])
            n267 = Build Array(w407, w409, w394, w393, w396) -> (w412:dbl[][])
            n268 = Build Array("Time (s)" ("element"), "Stage position (mm)" ("element"), "Force (N)" ("element"), "Roller position (mm)" ("element"), "V* (V)" ("element")) -> (w398:string[])
            n269 = Strip Path(path=w383) -> (stripped path=w384:path, name=w387:string)
            n270 = Transpose 2D Array(2D array=w412) -> (transposed array=w410:dbl[][])
            n271 = Concatenate Strings(w387, ".txt" ("name or relative path")) -> (w385:string)
            n272 = Array To Spreadsheet String(array=w398, 3:"%s") -> (spreadsheet string=w401:string)  [unwired: 1 in]
            n273 = local write "Pause Button"(TRUE) -> ()
            n274 = local write "Stop Test"(TRUE) -> ()
            n275 = Build Path(base path=w384, name or relative path=w385) -> (appended path=w381:path)
            "path" <- w381
            n276 = Open/Create/Replace File(file path (use dialog)=w381, operation (0:open)=T9."replace or create with confirmation") -> (refnum out=w382:refnum<file>, error out=w416:errorcluster)  [unwired: 4 in, 1 out]
            n277 = Array To Spreadsheet String(array=w410, 3:"%g" ("format string")) -> (spreadsheet string=w400:string)  [unwired: 1 in]
            n278 = Concatenate Strings(w401, w400) -> (w399:string)
            n279 = Write to Text File(file (use dialog)=w382, text=w399, error in=w416) -> (refnum out=w414:refnum<file>, error out=w415:errorcluster)  [unwired: 2 out]
            n280 = Close File(refnum=w414, error in=w415) -> ()  [unwired: 2 out]
          }
          frame #1 {
            n281 = local read "Save Results"() -> (w418:bool)
            n282 = case shown="True" w418 {
              frame False {
              }
              frame True {
                n283 = Get Date/Time In Seconds() -> (seconds since 1Jan1904=w429:timestamp)
                n284 = local read "Contact force (N):"() -> (w426:fxp<+/-,20,7>)
                n285 = local read "Travel distance (mm):"() -> (w424:dbl)
                n286 = local read "Stage speed (mm/s):"() -> (w423:dbl)
                n287 = local read "path"() -> (w435:path)
                n288 = local read "Start dwell time (s):"() -> (w422:dbl)
                n289 = local read "Stop dwell time (s):"() -> (w421:dbl)
                n290 = Get Date/Time String(seconds (now)=w429) -> (date string=w428:string, time string=w427:string)  [unwired: 2 in]
                n291 = Build Array(w428, w427) -> (w430:string[])
                n292 = Strip Path(path=w435) -> (stripped path=w441:path, name=w440:string)
                n293 = To Double Precision Float(number=w426) -> (double precision float=w425:dbl)
                n294 = Array To Spreadsheet String(array=w430, 3:"%s") -> (spreadsheet string=w431:string)  [unwired: 1 in]
                n295 = Build Array("Setpoint force (N)" ("element"), "Travel distance (mm)" ("element"), "Stage speed (mm/s)" ("element"), "Start dwell time (s)" ("element"), "Stop dwell time (s)" ("element")) -> (w444:string[])
                n296 = Build Array(w425, w424, w423, w422, w421) -> (w420:dbl[])
                n297 = Build Array(w420) -> (w419:dbl[][])
                n298 = Search and Replace String(input string=w440, search string=".txt" ("name or relative path"), replace string="_params.txt" ("name or relative path")) -> (result string=w438:string)  [unwired: 5 in, 3 out]
                n299 = Array To Spreadsheet String(array=w444, 3:"%s") -> (spreadsheet string=w451:string)  [unwired: 1 in]
                n300 = Array To Spreadsheet String(array=w419, 3:"%g" ("format string")) -> (spreadsheet string=w452:string)  [unwired: 1 in]
                n301 = Build Path(base path=w441, name or relative path=w438) -> (appended path=w436:path)
                n302 = Open/Create/Replace File(file path (use dialog)=w436, operation (0:open)=T9."replace or create with confirmation") -> (refnum out=w454:refnum<file>, error out=w443:errorcluster)  [unwired: 4 in, 1 out]
                n303 = Concatenate Strings(w451, w452) -> (w433:string)
                n304 = Concatenate Strings(w431, w433) -> (w432:string)
                n305 = Write to Text File(file (use dialog)=w454, text=w432, error in=w443) -> (refnum out=w456:refnum<file>, error out=w442:errorcluster)  [unwired: 2 out]
                n306 = Close File(refnum=w456, error in=w442) -> ()  [unwired: 2 out]
              }
            }
          }
          frame #2 {
            n307 = local write "Save As Button"(FALSE ("Pause Button")) -> ()
            n308 = local write "Save Results"(FALSE ("Save Results")) -> ()
          }
        }
      }
      event "Clear Button": Value Change {
        # "When the Clear button is pressed, all data are erased."
        n309 = event-data() -> ()  [unwired: 1 in, 1 out]
        n310 = local write "Pause Button"(TRUE) -> ()
      }
    }
    n311 = case shown="Error" w33 {
      tunnel: [w36 TRUE ("Discard?")] -> w34
      tunnel: w35 -> [w36 _]
      tunnel: w31 -> [_ w37]
      frame No Error {
      }
      frame Error {
        # "On error, send Exit message, and stop loop."
        n312 = call "Enqueue Message.vi"("Priority Message? (F)"=TRUE ("Discard?"), "Message"="Exit", "Message Queue"=w37) -> ()  [unwired: 7 in, 2 out]
      }
    }
  }
  n313 = while {
    tunnel: w11 -> [w465]
    tunnel: w19 -> [w470]
    shift-right: [w460] -> w23
    shift-left: w16 -> [w469]
    shift-right: [w463] -> _
    shift-left: T7 {"Switch to Safe State Ref"=refnum, "Run Manual Ref"=refnum, "Stop Manual Ref"=refnum, "Run Control Ref"=refnum, "Stop Control Ref"=refnum, "Update Control Configurations Ref"=refnum, "Ch 0 Setpoint Ref"=refnum, "Ch 1 Setpoint Ref"=refnum, "Ch 2 Setpoint Ref"=refnum, "Ch 3 Setpoint Ref"=refnum, "Ch 0 Manual Ref"=refnum, "Ch 1 Manual Ref"=refnum, "Ch 2 Manual Ref"=refnum, "Ch 3 Manual Ref"=refnum, "Control Configurations Ref"=refnum, "Custom Controller Cluster Ref"=refnum, "Control period (ticks) Ref"=refnum, "Roller control"=refnum, "Disable roller control"=refnum, "Test control"=refnum, "Disable test control"=refnum, "Controller Calcs"=refnum, "Observer Calcs"=refnum, "Other Calcs"=refnum} ("Measurement UI Controls") -> [w464]
    stop <- w471 stop-if-true
    # "UI Message Loop"
    n314 = call "Dequeue Message.vi"("error in (no error)"=w469, "Message Queue"=w465) -> ("error out"=w468:errorcluster, "Message Data"=w466:variant, "Message"=w467:string, "dup Message Queue"=w462:refnum<queue>)  [unwired: 6 in]
    n315 = case "Message Cases" shown="\"Disable Controls\"" w467 {
      selector: w467 -> [_ _ _ _ _ _ _ _ _ w621 _ _ _ _ w687 _ w753 _ _ _ _ _ _ _ _ _ w886]
      tunnel: w462 -> [w473 w488 _ _ w561 _ w579 _ w597 w622 _ _ _ _ _ _ w757 _ _ _ _ _ _ _ w871 _ _]
      tunnel: w468 -> [w475 w506 w535 w545 w566 w577 w581 w586 w617 w624 w642 w653 w664 w675 w688 w712 w767 w788 w798 w810 w820 w834 w846 w857 w876 w881 _]
      tunnel: [w474 w489 w535 w545 w560 w577 w580 w585 w600 w623 w641 w652 w663 w674 w689 w711 w768 w786 w796 w809 w819 w833 w845 w858 w877 w880 w884] -> w461
      tunnel: [_ _ _ _ _ _ _ _ _ _ _ _ _ _ _ _ _ _ _ _ _ _ _ _ TRUE _ _] -> w471
      tunnel: w466 -> [_ _ _ _ _ _ _ _ w615 _ _ _ _ w676 w686 w710 w765 w785 w797 w808 w821 w831 w843 w856 _ _ _]
      tunnel: w470 -> [_ _ _ _ _ _ _ _ _ _ _ _ _ _ _ _ _ _ _ _ _ _ _ _ w875 _ _]
      tunnel: w464 -> [w476 w505 w534 w556 w565 w576 w583 w587 w612 w625 w643 w654 w665 w677 w690 w709 w769 w787 w799 w811 w823 w835 w847 w859 w873 w879 w882]
      tunnel: [w476 w504 w534 w556 w565 w576 w583 w587 w612 w625 w643 w654 w665 w677 w690 w709 w769 w787 w799 w811 w823 w835 w847 w859 w873 w879 w882] -> w463
      frame "Initialize" {
        # "Initialize - Send 'Initialize UI Refs' message to get the UI references bundled and initialized appropriately."
        n316 = call "Enqueue Message.vi"("error in (no error)"=w475, "Message"="Initialize UI Refs", "Message Queue"=w473) -> ("error out"=w474:errorcluster)  [unwired: 7 in, 1 out]
      }
      frame "Initialize UI Refs" {
        # "Send a message to disable them all, since there is no connection at the start."
        # "Initialize UI Refs - Bundle up a cluster of references of all UI elements that are programmatically manipulated."
        n317 = control-ref of="Switch to Safe State"() -> (w503:refnum<vi>)
        n318 = control-ref of="Run Manual"() -> (w502:refnum<vi>)
        n319 = control-ref of="Stop Manual"() -> (w501:refnum<vi>)
        n320 = control-ref of="Run Control"() -> (w500:refnum<vi>)
        n321 = control-ref of="Stop Control"() -> (w499:refnum<vi>)
        n322 = control-ref of="Update Control Configuration"() -> (w498:refnum<vi>)
        n323 = control-ref of="Roller control"() -> (w483:refnum<vi>)
        n324 = control-ref of="Disable roller control"() -> (w482:refnum<vi>)
        n325 = control-ref of="Test control"() -> (w481:refnum<vi>)
        n326 = control-ref of="Disable test control"() -> (w480:refnum<vi>)
        n327 = control-ref of="Observer Calcs"() -> (w478:refnum<vi>)
        n328 = control-ref of="Controller Calcs"() -> (w479:refnum<vi>)
        n329 = control-ref of="Other Calcs"() -> (w477:refnum<vi>)
        n330 = control-ref of="Control period (ticks)"() -> (w484:refnum<vi>)
        n331 = control-ref of="Other Controller Gains"() -> (w485:refnum<vi>)
        n332 = control-ref of="Custom Controller Inputs"() -> ()  [unwired: 1 out]
        n333 = control-ref of="Channel 0 Setpoint"() -> (w497:refnum<vi>)
        n334 = control-ref of="Channel 1 Setpoint"() -> (w496:refnum<vi>)
        n335 = control-ref of="Channel 2 Setpoint"() -> (w495:refnum<vi>)
        n336 = control-ref of="Channel 3 Setpoint"() -> (w494:refnum<vi>)
        n337 = control-ref of="Channel 0 Manual Value"() -> (w493:refnum<vi>)
        n338 = control-ref of="Channel 1 Manual Value"() -> (w492:refnum<vi>)
        n339 = control-ref of="Channel 2 Manual Value"() -> (w491:refnum<vi>)
        n340 = control-ref of="Channel 3 Manual Value"() -> (w490:refnum<vi>)
        n341 = control-ref of="Control Configurations"() -> (w486:refnum<vi>)
        n342 = call "Enqueue Message.vi"("error in (no error)"=w506, "Message"="Disable Controls", "Message Queue"=w488) -> ("error out"=w489:errorcluster)  [unwired: 7 in, 1 out]
        n343 = Bundle By Name(cluster=w505, "Switch to Safe State Ref"=w503, "Run Manual Ref"=w502, "Stop Manual Ref"=w501, "Run Control Ref"=w500, "Stop Control Ref"=w499, "Update Control Configurations Ref"=w498, "Ch 0 Setpoint Ref"=w497, "Ch 1 Setpoint Ref"=w496, "Ch 2 Setpoint Ref"=w495, "Ch 3 Setpoint Ref"=w494, "Ch 0 Manual Ref"=w493, "Ch 1 Manual Ref"=w492, "Ch 2 Manual Ref"=w491, "Ch 3 Manual Ref"=w490, "Control Configurations Ref"=w486, "Custom Controller Cluster Ref"=w485, "Control period (ticks) Ref"=w484, "Roller control"=w483, "Disable roller control"=w482, "Test control"=w481, "Disable test control"=w480, "Controller Calcs"=w479, "Observer Calcs"=w478, "Other Calcs"=w477) -> (w504:T7)
      }
      frame "Disable Controls" {
        w516 = 0
        # "With the control options disabled, the only thing the user can do is Connect. Make sure the IP address string and connect button are enabled."
        # "Disable All Controls - Set all controls in the UI Refs cluster to \"Disabled and Grayed Out\"."
        n344 = Unbundle(w534) -> ("Switch to Safe State Ref"=w533:refnum<vi>, "Run Manual Ref"=w532:refnum<vi>, "Stop Manual Ref"=w531:refnum<vi>, "Run Control Ref"=w530:refnum<vi>, "Stop Control Ref"=w529:refnum<vi>, "Update Control Configurations Ref"=w528:refnum<vi>, "Ch 0 Setpoint Ref"=w527:refnum<vi>, "Ch 1 Setpoint Ref"=w526:refnum<vi>, "Ch 2 Setpoint Ref"=w525:refnum<vi>, "Ch 3 Setpoint Ref"=w524:refnum<vi>, "Ch 0 Manual Ref"=w523:refnum<vi>, "Ch 1 Manual Ref"=w522:refnum<vi>, "Ch 2 Manual Ref"=w521:refnum<vi>, "Ch 3 Manual Ref"=w520:refnum<vi>, "Control Configurations Ref"=w519:refnum<vi>, "Custom Controller Cluster Ref"=w515:refnum<vi>, "Control period (ticks) Ref"=w514:refnum<vi>, "Roller control"=w513:refnum<vi>, "Disable roller control"=w512:refnum<vi>, "Test control"=w511:refnum<vi>, "Disable test control"=w510:refnum<vi>, "Controller Calcs"=w509:refnum<vi>, "Observer Calcs"=w508:refnum<vi>, "Other Calcs"=w507:refnum<vi>)
        n345 = Build Array(w533, w532, w531, w530, w529, w528, w527, w526, w525, w524, w523, w522, w521, w520, w519, w515, w514, w513, w512, w511, w510, w509, w508, w507) -> (w518:refnum<vi>[])
        n346 = call "Set Enable State on Multiple Controls.vi"("Enable?"=FALSE, "Controls"=w518) -> ()  [unwired: 10 in]
        n347 = property on="Controller Address" class="Str"("DisabledEnum"=w516) -> ()  [unwired: 2 in, 2 out]
        n348 = property on="Connect to Controller" class="Bool"("DisabledEnum"=w516) -> ()  [unwired: 2 in, 2 out]
      }
      frame "Enable Configuration Controls" {
        w557 = 2
        # "Once connected, the user shouldn't be able to change the connection settings unless he gets disconnected."
        # "Enable Configuration Controls - After successful connection, ensure appropriate controls are enabled."
        n349 = Unbundle By Name(w556) -> ("Update Control Configurations Ref"=w555:refnum<vi>, "Ch 0 Setpoint Ref"=w554:refnum<vi>, "Ch 1 Setpoint Ref"=w553:refnum<vi>, "Ch 2 Setpoint Ref"=w552:refnum<vi>, "Ch 3 Setpoint Ref"=w551:refnum<vi>, "Ch 0 Manual Ref"=w550:refnum<vi>, "Ch 1 Manual Ref"=w549:refnum<vi>, "Ch 2 Manual Ref"=w548:refnum<vi>, "Ch 3 Manual Ref"=w547:refnum<vi>, "Control Configurations Ref"=w546:refnum<vi>, "Custom Controller Cluster Ref"=w544:refnum<vi>, "Control period (ticks) Ref"=w543:refnum<vi>, "Roller control"=w542:refnum<vi>, "Disable roller control"=w541:refnum<vi>, "Test control"=w540:refnum<vi>, "Disable test control"=w539:refnum<vi>, "Controller Calcs"=w538:refnum<vi>, "Observer Calcs"=w537:refnum<vi>, "Other Calcs"=w536:refnum<vi>)
        n350 = Build Array(w555, w554, w553, w552, w551, w550, w549, w548, w547, w546, w544, w543, w542, w541, w540, w539, w538, w537, w536) -> (w559:refnum<vi>[])
        n351 = call "Set Enable State on Multiple Controls.vi"("Enable?"=TRUE, "Controls"=w559) -> ()  [unwired: 10 in]
        n352 = property on="Controller Address" class="Str"("DisabledEnum"=w557) -> ()  [unwired: 2 in, 2 out]
        n353 = property on="Connect to Controller" class="Bool"("DisabledEnum"=w557) -> ()  [unwired: 2 in, 2 out]
      }
      frame "Connect" {
        # "Connect - Attempt to connect to both streams, and the variables, on the RT target."
        n354 = call "UI - Initiate Connection.vi"("error in (no error)"=w566, "Controller Address"="Controller Address", "Message Queue"=w561) -> ("error out"=w563:errorcluster, "Connected?"=w562:bool)  [unwired: 7 in]
        "Connected?" <- w562
        n355 = case shown="True" w562 {
          tunnel: w563 -> [w567 w571]
          tunnel: w561 -> [_ w570]
          tunnel: [w567 w569] -> w560
          frame False {
          }
          frame True {
            n356 = call "Enqueue Message.vi"("error in (no error)"=w571, "Message"="Enable Configuration Controls", "Message Queue"=w570) -> ("error out"=w569:errorcluster)  [unwired: 7 in, 1 out]
          }
        }
      }
      frame "Close Connections" {
        # "Close Connections - Close the connections shared with the Monitoring Loop."
        n357 = global read "Global - UI Stream and Variable Connections.vi" "UI Command Stream"() -> (w575:refnum<k21>)
        n358 = global read "Global - UI Stream and Variable Connections.vi" "RT Message Stream"() -> (w574:refnum<k21>)
        n359 = global read "Global - UI Stream and Variable Connections.vi" "Variable References"() -> (w573:T12)
        n360 = local write "Connected?"(FALSE ("Connected?")) -> ()
        n361 = Destroy Stream Endpoint(11:w575) -> ()  [unwired: 1 in, 1 out]
        n362 = Destroy Stream Endpoint(11:w574) -> ()  [unwired: 1 in, 1 out]
        n363 = call "Close Variable Connections.vi"("Variable References"=w573) -> ()  [unwired: 11 in]
      }
      frame "Disconnect UI" {
        # "Disconnect UI - Something has gone wrong with the connection. Reinitialize the UI to its disconnected state."
        n364 = local write "Connected?"(FALSE ("Connected?")) -> ()
        n365 = call "Enqueue Message.vi"("error in (no error)"=w581, "Message"="Disable Controls", "Message Queue"=w579) -> ("error out"=w580:errorcluster)  [unwired: 7 in, 1 out]
      }
      frame "Get Settings from FPGA" {
        # "Get Settings from FPGA - Send a command to the RT to retrieve all current FPGA Main VI parameter values and send them back to the UI."
        n366 = local read "Connected?"() -> (w584:bool)
        n367 = case shown="True" w584 {
          tunnel: w586 -> [w588 w592]
          tunnel: [w588 w591] -> w585
          frame False {
            # "Don't bother trying to send a message to the RT system if UI Main VI isn't even connected"
          }
          frame True {
            n368 = global read "Global - UI Stream and Variable Connections.vi" "UI Command Stream"() -> (w589:refnum<k21>)
            n369 = shared-variable-write(w589, w592, T18 {"Message"="Send FPGA Configuration to UI", "Message Data"=variant} ("data in")) -> (w591:errorcluster)  [unwired: 1 in, 2 out]
          }
        }
      }
      frame "Initial UI Values" {
        # "Initial UI Values - These are the current values of the FPGA Main VI's R/W controls. They are used to initialize the panel of UI Main VI upon successful connection to the RT target."
        # "Set values of all manual and setpoint controls via reference."
        n370 = Variant To Data(error in=w617, type=T19 {"FPGA State"=enum."Safe State", "Manual Values"={"Channel 0"=0.0, "Channel 1"=0.0, "Channel 2"=0.0, "Channel 3"=0.0}, "Setpoints"={"Channel 0"=0.0, "Channel 1"=0.0, "Channel 2"=0.0, "Channel 3"=0.0}, "Control Configurations"=[]} ("All FPGA Configuration Values"), Variant=w615) -> (data=w613:T19, error out=w616:errorcluster)
        n371 = Unbundle By Name(w612) -> ("Ch 0 Setpoint Ref"=w611:refnum<vi>, "Ch 1 Setpoint Ref"=w610:refnum<vi>, "Ch 2 Setpoint Ref"=w609:refnum<vi>, "Ch 3 Setpoint Ref"=w608:refnum<vi>, "Ch 0 Manual Ref"=w607:refnum<vi>, "Ch 1 Manual Ref"=w606:refnum<vi>, "Ch 2 Manual Ref"=w605:refnum<vi>, "Ch 3 Manual Ref"=w604:refnum<vi>)
        n372 = Unbundle By Name(w613) -> ("Setpoints"=w595:T13, "Manual Values"=w593:T13, "Control Configurations"=w601:T5[], "FPGA State"=w598:T20)
        n373 = Build Array(w611, w610, w609, w608, w607, w606, w605, w604) -> (w603:refnum<vi>[])
        n374 = To Variant(anything=w593) -> (Variant=w594:variant)
        n375 = To Variant(anything=w595) -> (Variant=w596:variant)
        n376 = local write "Current FPGA Control Mode"(w598) -> ()
        n377 = Build Array(w596, w594) -> (w602:variant[])
        n378 = local write "Control Configurations"(w601) -> ()
        n379 = for {
          tunnel: w603 -> [w619] mode=indexing
          tunnel: w602 -> [w618] mode=indexing
          n380 = property class="DigNum"(reference=w619, "Value"=w618) -> ()  [unwired: 1 in, 2 out]
        }
        n381 = call "Enqueue Message.vi"("error in (no error)"=w616, "Message Data"=w598, "Message"="Update Display Mode", "Message Queue"=w597) -> ("error out"=w600:errorcluster)  [unwired: 6 in, 1 out]
      }
      frame "Run Control", "Run Manual", "Run Safe State", "Stop Control", "Stop Manual" {
        # "Run/Stop buttons - Send a command to switch the FPGA into the appropriate state. Send a message to update this UI to reflect the new state."
        n382 = local read "Connected?"() -> (w620:bool)
        n383 = case shown="True" w620 {
          tunnel: w624 -> [w626 w636]
          tunnel: [w626 w632] -> w623
          tunnel: w622 -> [_ w631]
          tunnel: w621 -> [_ w630]
          frame False {
            # "Don't bother trying to send a message to the RT system if UI Main VI isn't even connected"
          }
          frame True {
            # "Run Manual and Run Control switch into their respective states. Anything else switches to Safe State."
            n384 = case shown="\"Run Control\"" w630 {
              tunnel: [FPGA_State."Safe State" ("FPGA State") FPGA_State."Control (PID)" ("FPGA State") FPGA_State."Manual" ("FPGA State")] -> w627
              frame "Safe State", "Stop Control", "Stop Manual", Default {
              }
              frame "Run Control" {
              }
              frame "Run Manual" {
              }
            }
            n385 = global read "Global - UI Stream and Variable Connections.vi" "UI Command Stream"() -> (w628:refnum<k21>)
            n386 = Bundle("Update FPGA State", "FPGA State"=w627) -> (w633:cluster{string, "FPGA State":T20})  [unwired: 1 in]
            n387 = shared-variable-write(w628, w636, w633) -> (w635:errorcluster)  [unwired: 1 in, 2 out]
            n388 = call "Enqueue Message.vi"("error in (no error)"=w635, "Message Data"=w627, "Message"="Update Display Mode", "Message Queue"=w631) -> ("error out"=w632:errorcluster)  [unwired: 6 in, 1 out]
          }
        }
      }
      frame "Update Control period" {
        n389 = local read "Connected?"() -> (w640:bool)
        n390 = case shown="True" w640 {
          tunnel: w642 -> [w644 w650]
          tunnel: [w644 w649] -> w641
          frame False {
            # "Don't bother trying to send a message to the RT system if UI Main VI isn't even connected"
          }
          frame True {
            n391 = global read "Global - UI Stream and Variable Connections.vi" "UI Command Stream"() -> (w646:refnum<k21>)
            n392 = local read "Control period (ticks)"() -> (w645:u32)
            n393 = Bundle("Update Control period", "Control period (ticks)"=w645) -> (w647:cluster{string, "Control period (ticks)":u32})  [unwired: 1 in]
            n394 = shared-variable-write(w646, w650, w647) -> (w649:errorcluster)  [unwired: 1 in, 2 out]
          }
        }
      }
      frame "Update Control Configuration" {
        # "Update Control Configuration - Send all control configurations to RT to be sent down to the FPGA."
        n395 = local read "Connected?"() -> (w651:bool)
        n396 = case shown="True" w651 {
          tunnel: w653 -> [w655 w661]
          tunnel: [w655 w660] -> w652
          frame False {
            # "Don't bother trying to send a message to the RT system if UI Main VI isn't even connected"
          }
          frame True {
            n397 = global read "Global - UI Stream and Variable Connections.vi" "UI Command Stream"() -> (w656:refnum<k21>)
            n398 = Bundle("Update Control Configurations", "Control Configurations"="Control Configurations") -> (w658:cluster{string, "Control Configurations":T5[]})  [unwired: 1 in]
            n399 = shared-variable-write(w656, w661, w658) -> (w660:errorcluster)  [unwired: 1 in, 2 out]
          }
        }
      }
      frame "Update Custom Controller" {
        # "Update Control Configuration - Send all control configurations to RT to be sent down to the FPGA."
        n400 = local read "Connected?"() -> (w662:bool)
        n401 = case shown="True" w662 {
          tunnel: w664 -> [w666 w672]
          tunnel: [w666 w671] -> w663
          frame False {
            # "Don't bother trying to send a message to the RT system if UI Main VI isn't even connected"
          }
          frame True {
            n402 = global read "Global - UI Stream and Variable Connections.vi" "UI Command Stream"() -> (w668:refnum<k21>)
            n403 = Bundle("Update Custom Controller", "Custom Controller Inputs"="Custom Controller Inputs") -> (w669:cluster{string, "Custom Controller Inputs":T6})  [unwired: 1 in]
            n404 = shared-variable-write(w668, w672, w669) -> (w671:errorcluster)  [unwired: 1 in, 2 out]
          }
        }
      }
      frame "Update stage speed" {
        n405 = local read "Connected?"() -> (w673:bool)
        n406 = case shown="True" w673 {
          tunnel: w675 -> [w678 w684]
          tunnel: [w678 w683] -> w674
          tunnel: w676 -> [_ w679]
          frame False {
            # "Don't bother trying to send a message to the RT system if UI Main VI isn't even connected"
          }
          frame True {
            n407 = global read "Global - UI Stream and Variable Connections.vi" "UI Command Stream"() -> (w680:refnum<k21>)
            n408 = Bundle("Update stage speed", "Message Data"=w679) -> (w681:cluster{string, "Message Data":variant})  [unwired: 1 in]
            n409 = shared-variable-write(w680, w684, w681) -> (w683:errorcluster)  [unwired: 1 in, 2 out]
          }
        }
      }
      frame "Update Manual Values", "Update Setpoints" {
        # "Update Manual Values/Setpoints - Send all manual values/setpoints to RT to be sent down to the FPGA."
        n410 = local read "Connected?"() -> (w685:bool)
        n411 = case shown="True" w685 {
          tunnel: [w691 w697] -> w689
          tunnel: w688 -> [w691 w695]
          tunnel: w687 -> [_ w694]
          tunnel: w686 -> [_ w693]
          frame False {
            # "Don't bother trying to send a message to the RT system if UI Main VI isn't even connected"
          }
          frame True {
            n412 = global read "Global - UI Stream and Variable Connections.vi" "UI Command Stream"() -> (w692:refnum<k21>)
            n413 = Bundle(w694, "Message Data"=w693) -> (w696:cluster{string, "Message Data":variant})  [unwired: 1 in]
            n414 = shared-variable-write(w692, w695, w696) -> (w697:errorcluster)  [unwired: 1 in, 2 out]
          }
        }
      }
      frame "Update Display Mode" {
        # "Update Display Mode - Enable/Disable Controls appropriately for the new display mode."
        n415 = Variant To Data(error in=w712, type=FPGA_State."Safe State" ("FPGA State"), Variant=w710) -> (data=w708:T20, error out=w711:errorcluster)
        n416 = Unbundle By Name(w709) -> ("Switch to Safe State Ref"=w707:refnum<vi>, "Run Manual Ref"=w706:refnum<vi>, "Stop Manual Ref"=w705:refnum<vi>, "Run Control Ref"=w704:refnum<vi>, "Stop Control Ref"=w703:refnum<vi>, "Roller control"=w701:refnum<vi>, "Disable roller control"=w700:refnum<vi>, "Test control"=w699:refnum<vi>, "Disable test control"=w698:refnum<vi>)
        n417 = case shown="\"Safe State\"" w708 {
          tunnel: w707 -> [w721 w734 w745]
          tunnel: w706 -> [w717 w733 w747]
          tunnel: w705 -> [w720 w732 w744]
          tunnel: w704 -> [w719 w730 w746]
          tunnel: w703 -> [w718 w731 w743]
          tunnel: w701 -> [w715 w729 w742]
          tunnel: w700 -> [w714 w728 w741]
          tunnel: w699 -> [w716 w727 w740]
          tunnel: w698 -> [w713 w726 w739]
          frame "Control (PID)" {
            n418 = Build Array "Controls to Enable"(w721, w718, w717, w715, w713) -> (w725:refnum<vi>[])
            n419 = Build Array "Controls to Disable"(w720, w719, w716, w714) -> (w723:refnum<vi>[])
            n420 = call "Set Enable State on Multiple Controls.vi"("Enable?"=FALSE, "Controls"=w723) -> ()  [unwired: 10 in]
            n421 = call "Set Enable State on Multiple Controls.vi"("Enable?"=TRUE, "Controls"=w725) -> ()  [unwired: 10 in]
          }
          frame "Manual" {
            n422 = Build Array "Controls to Enable"(w734, w732, w730, w728, w727) -> (w738:refnum<vi>[])
            n423 = Build Array "Controls to Disable"(w733, w731, w729, w726) -> (w736:refnum<vi>[])
            n424 = call "Set Enable State on Multiple Controls.vi"("Enable?"=FALSE, "Controls"=w736) -> ()  [unwired: 10 in]
            n425 = call "Set Enable State on Multiple Controls.vi"("Enable?"=TRUE, "Controls"=w738) -> ()  [unwired: 10 in]
          }
          frame "Safe State" {
            # "This frame runs when FPGA is in Safe State. Only enable the two run buttons."
            n426 = Build Array "Controls to Enable"(w747, w746, w742, w740) -> (w751:refnum<vi>[])
            n427 = Build Array "Controls to Disable"(w745, w744, w743, w741, w739) -> (w749:refnum<vi>[])
            n428 = call "Set Enable State on Multiple Controls.vi"("Enable?"=FALSE, "Controls"=w749) -> ()  [unwired: 10 in]
            n429 = call "Set Enable State on Multiple Controls.vi"("Enable?"=TRUE, "Controls"=w751) -> ()  [unwired: 10 in]
          }
        }
      }
      frame "Critical Error", "Log-Only Error", "Non-Critical Error", "RT Error" {
        # "Error - Display message in status indicator on panel.  If it's a critical error, shut down this VI with an 'Exit' message."
        n430 = case shown="Default" w753 {
          selector: w753 -> [_ w771]
          tunnel: ["UI Error" w771] -> w752
          frame Default {
          }
          frame "RT Error" {
          }
        }
        n431 = Variant To Data(error in=w767, type=errorcluster {"status"=FALSE, "code"=0, "source"=""} ("error constant"), Variant=w765) -> (data=w760:errorcluster, error out=w766:errorcluster)
        n432 = Unbundle By Name(w760) -> ("code"=w759:i32, "source"=w763:string)
        n433 = Format Date/Time String() -> (date/time string=w762:string)  [unwired: 3 in]
        n434 = Format Into String(format string="\n%s: %s %d - %s", w762, w752, w759, w763) -> (resulting string=w754:string)  [unwired: 2 in, 1 out]
        n435 = call "Enqueue Message.vi"("error in (no error)"=w766, "Message Data"=w754, "Message"="Update System Status", "Message Queue"=w757) -> ("error out"=w758:errorcluster, "dup Message Queue"=w756:refnum<queue>)  [unwired: 6 in]
        n436 = case shown="Default" w753 {
          tunnel: w758 -> [w772 w776]
          tunnel: w756 -> [_ w774]
          tunnel: [w772 w775] -> w768
          frame Default {
          }
          frame "Critical Error" {
            n437 = call "Enqueue Message.vi"("error in (no error)"=w776, "Message"="Exit", "Message Queue"=w774) -> ("error out"=w775:errorcluster)  [unwired: 7 in, 1 out]
          }
        }
      }
      frame "Update System Status" {
        # "Code Recommended - The code below ensures that the System Status string value does not become too large.  It uses the same maximum size as the RT error log to determine whether or not to remove the last half of the log string. Change this logic if you wish to maintain more/less of the information in the System Status string."
        # "Update System Status - Add a new string to the beginning of the System Status string on the UI."
        n438 = Variant To Data(error in=w788, type="", Variant=w785) -> (data=w782:string, error out=w786:errorcluster)
        n439 = local read "System Status"() -> (w780:string)
        n440 = global read "Global - Configuration Options.vi" "Error Log Max Size (bytes)"() -> (w778:i64)
        n441 = String Length(string=w780) -> (length=w781:i32)
        n442 = Greater?(x=w781, y=w778) -> (0:w779:bool)
        n443 = case shown="True" w779 {
          tunnel: w780 -> [w789 w793]
          tunnel: w778 -> [_ w792]
          tunnel: [w789 w794] -> w777
          frame False {
          }
          frame True {
            n444 = Divide(x=w792, y=i64 2) -> (x/y=w791:dbl)
            n445 = String Subset(string=w793, length (rest)=w791) -> (substring=w794:string)  [unwired: 1 in]
          }
        }
        n446 = Concatenate Strings(w782, w777) -> (→"System Status":string)
      }
      frame "Home roller" {
        n447 = local read "Connected?"() -> (w795:bool)
        n448 = case shown="True" w795 {
          tunnel: [w800 w806] -> w796
          tunnel: w798 -> [w800 w804]
          tunnel: w797 -> [_ w803]
          frame False {
            # "Don't bother trying to send a message to the RT system if UI Main VI isn't even connected"
          }
          frame True {
            n449 = global read "Global - UI Stream and Variable Connections.vi" "UI Command Stream"() -> (w802:refnum<k21>)
            n450 = Bundle("Message"="Update Manual Values", "Message Data"=w803) -> (w805:T18)  [unwired: 1 in]
            n451 = shared-variable-write(w802, w804, w805) -> (w806:errorcluster)  [unwired: 1 in, 2 out]
          }
        }
      }
      frame "Contact roller" {
        n452 = local read "Connected?"() -> (w807:bool)
        n453 = case shown="True" w807 {
          tunnel: [w812 w818] -> w809
          tunnel: w810 -> [w812 w816]
          tunnel: w808 -> [_ w815]
          frame False {
            # "Don't bother trying to send a message to the RT system if UI Main VI isn't even connected"
          }
          frame True {
            n454 = global read "Global - UI Stream and Variable Connections.vi" "UI Command Stream"() -> (w814:refnum<k21>)
            n455 = Bundle("Message"="Update Manual Values", "Message Data"=w815) -> (w817:T18)  [unwired: 1 in]
            n456 = shared-variable-write(w814, w816, w817) -> (w818:errorcluster)  [unwired: 1 in, 2 out]
          }
        }
      }
      frame "Stop roller" {
        n457 = local read "Connected?"() -> (w822:bool)
        n458 = case shown="True" w822 {
          tunnel: [w824 w830] -> w819
          tunnel: w820 -> [w824 w828]
          tunnel: w821 -> [_ w827]
          frame False {
            # "Don't bother trying to send a message to the RT system if UI Main VI isn't even connected"
          }
          frame True {
            n459 = global read "Global - UI Stream and Variable Connections.vi" "UI Command Stream"() -> (w826:refnum<k21>)
            n460 = Bundle("Message"="Update Manual Values", "Message Data"=w827) -> (w829:T18)  [unwired: 1 in]
            n461 = shared-variable-write(w826, w828, w829) -> (w830:errorcluster)  [unwired: 1 in, 2 out]
          }
        }
      }
      frame "Home stage" {
        n462 = local read "Connected?"() -> (w832:bool)
        n463 = case shown="True" w832 {
          tunnel: w834 -> [w836 w842]
          tunnel: [w836 w841] -> w833
          tunnel: w831 -> [_ w837]
          frame False {
            # "Don't bother trying to send a message to the RT system if UI Main VI isn't even connected"
          }
          frame True {
            n464 = global read "Global - UI Stream and Variable Connections.vi" "UI Command Stream"() -> (w838:refnum<k21>)
            n465 = Bundle("Home stage", "Message Data"=w837) -> (w839:cluster{string, "Message Data":variant})  [unwired: 1 in]
            n466 = shared-variable-write(w838, w842, w839) -> (w841:errorcluster)  [unwired: 1 in, 2 out]
          }
        }
      }
      frame "Go stage" {
        n467 = local read "Connected?"() -> (w844:bool)
        n468 = case shown="True" w844 {
          tunnel: w846 -> [w848 w854]
          tunnel: [w848 w853] -> w845
          tunnel: w843 -> [_ w849]
          frame False {
            # "Don't bother trying to send a message to the RT system if UI Main VI isn't even connected"
          }
          frame True {
            n469 = global read "Global - UI Stream and Variable Connections.vi" "UI Command Stream"() -> (w850:refnum<k21>)
            n470 = Bundle("Go stage", "Message Data"=w849) -> (w851:cluster{string, "Message Data":variant})  [unwired: 1 in]
            n471 = shared-variable-write(w850, w854, w851) -> (w853:errorcluster)  [unwired: 1 in, 2 out]
          }
        }
      }
      frame "Stop stage" {
        n472 = local read "Connected?"() -> (w855:bool)
        n473 = case shown="True" w855 {
          tunnel: w857 -> [w860 w866]
          tunnel: [w860 w865] -> w858
          tunnel: w856 -> [_ w861]
          frame False {
            # "Don't bother trying to send a message to the RT system if UI Main VI isn't even connected"
          }
          frame True {
            n474 = global read "Global - UI Stream and Variable Connections.vi" "UI Command Stream"() -> (w862:refnum<k21>)
            n475 = Bundle("Stop stage", "Message Data"=w861) -> (w863:cluster{string, "Message Data":variant})  [unwired: 1 in]
            n476 = shared-variable-write(w862, w866, w863) -> (w865:errorcluster)  [unwired: 1 in, 2 out]
          }
        }
      }
      frame "Exit" {
        # "Close all connections"
        # "Stop Monitoring Loop"
        # "Stop Event Handling Loop"
        # "Release the UI Message queue reference"
        # "Stop UI Message Loop"
        # "Exit - Fire the User Event to stop the Event Handling Loop, and toggle the local variable to stop the Monitoring Loop.  This message alone causes all three loops to stop."
        n477 = global write "Global - All UI Loop Stop.vi" "All UI Loop Stop"(TRUE ("Stop Monitoring Loop")) -> ()
        n478 = call "Fire User Event - Stop.vi"("User Event - Stop"=w875) -> ("error out"=w874:errorcluster)  [unwired: 10 in]
        n479 = Release Queue(queue=w871, error in (no error)=w876) -> (error out=w872:errorcluster)  [unwired: 1 in, 2 out]
        n480 = global read "Global - UI Stream and Variable Connections.vi" "UI Command Stream"() -> (w869:refnum<k21>)
        n481 = global read "Global - UI Stream and Variable Connections.vi" "RT Message Stream"() -> (w868:refnum<k21>)
        n482 = global read "Global - UI Stream and Variable Connections.vi" "Variable References"() -> (w867:T12)
        n483 = Destroy Stream Endpoint(11:w869) -> ()  [unwired: 1 in, 1 out]
        n484 = Destroy Stream Endpoint(11:w868) -> ()  [unwired: 1 in, 1 out]
        n485 = call "Close Variable Connections.vi"("Variable References"=w867) -> ()  [unwired: 11 in]
        n486 = Merge Errors(w874, w872) -> (w877:errorcluster)
      }
      frame "---Copy This Frame---" {
        # "Duplicate this frame when creating new messages.  Change this comment in the duplicated frame to describe this message."
        n487 = Merge Errors(w881) -> (w880:errorcluster)
      }
      frame Default {
        # "'Default' case only runs if there is a message that isn't defined in any of the other cases.  Output a programming error."
        n488 = Format Into String(format string="The invalid message string \"%s\" was received in the Message Handling Loop." ("Invalid Message Loop Message"), w886) -> (resulting string=w883:string)  [unwired: 2 in, 1 out]
        n489 = call <vilib>:"Error Cluster From Error Code.vi"("error message (\"\")"=w883, "error code (0)"=1) -> ("error out"=w884:errorcluster)  [unwired: 7 in]
      }
    }
    n490 = call "UI Error Handler - Message Handler.vi"("error in (no error)"=w461, "Message Queue"=w462) -> ()  [unwired: 9 in, 1 out]
    n491 = call <vilib>:"Clear Errors.vi"("error in (no error)"=w461) -> ("error out"=w460:errorcluster)  [unwired: 6 in]
  }
  n492 = while {
    tunnel: w11 -> [w910]
    shift-right: [w903] -> _
    shift-left: dbl[] [] -> [w902]
    shift-right: [w901] -> _
    shift-left: dbl[] [] -> [w898]
    shift-right: [w900] -> _
    shift-left: dbl[] [] -> [w899]
    shift-right: [w897] -> _
    shift-left: dbl[] [] -> [w894]
    shift-right: [w896] -> _
    shift-left: dbl[] [] -> [w893]
    shift-right: [w895] -> _
    shift-left: dbl[] [] -> [w892]
    shift-right: [w889] -> _
    shift-left: dbl[] [] -> [w890]
    stop <- w911 stop-if-true
    (unwired) refnum<vi> refnum ("Controller Calculations")
    # "Only read monitoring variables if:\n1.The UI Main VI is \nconnected to the RT target\nAND\n2. The Pause button is not depressed\nAND\n3. The Save button is not depressed"
    # "Only the 'Exit' message in the UI Message Loop can stop the Monitoring Loop."
    # "Monitoring Loop"
    n493 = local read "Connected?"() -> (w908:bool)
    n494 = Not(x="Pause Button") -> (.not. x?=w905:bool)
    n495 = Divide(x=1000.0, y="Display frequency (Hz)") -> (x/y=w891:dbl)
    n496 = To Unsigned Long Integer(number=w891) -> (unsigned 32bit integer=w888:u32)
    n497 = global write "Global - Configuration Options.vi" "Monitoring Loop Rate (ms)"(w888) -> ()
    n498 = And(x=w908, y=w905) -> (x .and. y?=w906:bool)
    n499 = case shown="True" w906 {
      tunnel: w910 -> [_ w1064]
      tunnel: w891 -> [w928 w1059]
      tunnel: [w926 w1003] -> w903
      tunnel: w902 -> [w925 w1054]
      tunnel: [w921 w1001] -> w901
      tunnel: [w923 w1002] -> w900
      tunnel: w899 -> [w924 w1048]
      tunnel: w898 -> [w922 w1047]
      tunnel: [w919 w1000] -> w897
      tunnel: [w917 w999] -> w896
      tunnel: [w915 w998] -> w895
      tunnel: w894 -> [w920 w1040]
      tunnel: w893 -> [w918 w1039]
      tunnel: w892 -> [w916 w1038]
      tunnel: w891 -> [_ w1030]
      tunnel: w890 -> [w914 w985]
      tunnel: [w913 w980] -> w889
      frame False {
        n500 = local read "Clear Button"() -> (w912:bool)
        n501 = Wait (ms)(milliseconds to wait=w928) -> ()  [unwired: 1 out]
        n502 = Not(x=w912) -> (.not. x?=w927:bool)
        n503 = case shown="False" w927 {
          tunnel: [w942 w957] -> w926
          tunnel: w925 -> [w941 w957]
          tunnel: w924 -> [w940 w956]
          tunnel: [w939 w956] -> w923
          tunnel: w922 -> [w938 w955]
          tunnel: [w937 w955] -> w921
          tunnel: w920 -> [w936 w954]
          tunnel: [w935 w954] -> w919
          tunnel: w918 -> [w934 w953]
          tunnel: [w933 w953] -> w917
          tunnel: w916 -> [w932 w952]
          tunnel: [w931 w952] -> w915
          tunnel: w914 -> [w930 w951]
          tunnel: [w929 w951] -> w913
          frame False {
            n504 = stacked-sequence {
              tunnel: [dbl[] [] _] -> w942
              tunnel: w941 -> [_ _]
              tunnel: w940 -> [_ _]
              tunnel: [dbl[] [] _] -> w939
              tunnel: w938 -> [_ _]
              tunnel: [dbl[] [] _] -> w937
              tunnel: w936 -> [_ _]
              tunnel: [dbl[] [] _] -> w935
              tunnel: w934 -> [_ _]
              tunnel: [dbl[] [] _] -> w933
              tunnel: w932 -> [_ _]
              tunnel: [dbl[] [] _] -> w931
              tunnel: w930 -> [_ _]
              tunnel: [dbl[] [] _] -> w929
              frame #0 {
                # "Clear all arrays"
              }
              frame #1 {
                w950 = FALSE ("Clear Button")
                n505 = local write "Pause Button"(w950) -> ()
                n506 = local write "Clear Button"(w950) -> ()
              }
            }
          }
          frame True {
          }
        }
      }
      frame True {
        # "Build the array for plotting"
        # "Get the time data"
        # "Serialize the shared variable calls to simplify the scheduling performed by LabVIEW at runtime"
        n507 = global read "Global - UI Stream and Variable Connections.vi" "Variable References"() -> (w1062:T12)
        n508 = call "UI - Read Stream from RT.vi"("Message Queue"=w1064) -> ("error out"=w1070:errorcluster, "Message Received?"=w1060:bool, "dup Message Queue"=w1063:refnum<queue>)  [unwired: 8 in]
        n509 = case shown="False" w1060 {
          tunnel: w1059 -> [w1130 _]
          frame False {
            n510 = Wait (ms)(milliseconds to wait=w1130) -> ()  [unwired: 1 out]
          }
          frame True {
            # "If a message was received, immediately read again"
          }
        }
        n511 = Unbundle By Name(w1062) -> ("CPU Usage"=w1076:refnum<k21>, "Contiguous Memory"=w1075:refnum<k21>, "Input Values"=w1074:refnum<k21>, "Output Values"=w1073:refnum<k21>, "FPGA Mode"=w1072:refnum<k21>, "Actual Loop Period"=w1071:refnum<k21>, "Controller Calcs"=w967:refnum<k21>, "Observer Calcs"=w963:refnum<k21>, "Other Calcs"=w960:refnum<k21>)
        n512 = Divide(x=w1030, y=2.0) -> (x/y=w986:dbl)
        n513 = shared-variable-read(w1076, w1070) -> (w1069:errorcluster, →"CPU Usage (%)":dbl)  [unwired: 2 out]
        n514 = shared-variable-read(w1075, w1069) -> (w1068:errorcluster, →"Largest Contiguous Memory (bytes)":dbl)  [unwired: 2 out]
        n515 = shared-variable-read(w1074, w1068) -> (w1067:errorcluster, w1078:T13)  [unwired: 2 out]
        n516 = shared-variable-read(w1073, w1067) -> (w1066:errorcluster, w1077:T13)  [unwired: 2 out]
        n517 = shared-variable-read(w1072, w1066) -> (w1065:errorcluster, →"Current FPGA Control Mode":T20)  [unwired: 2 out]
        n518 = shared-variable-read(w1071, w1065) -> (w965:errorcluster, w1029:u32)  [unwired: 2 out]
        "Actual Loop Period (ticks)" <- w1029
        n519 = shared-variable-read(w967, w965) -> (w964:errorcluster, →"Controller Calcs":T4)  [unwired: 2 out]
        n520 = shared-variable-read(w963, w964) -> (w961:errorcluster, →"Observer Calcs":T3)  [unwired: 2 out]
        n521 = shared-variable-read(w960, w961) -> (w958:errorcluster, →"Other Calcs":T2)  [unwired: 2 out]
        n522 = To Double Precision Float(number=w1078) -> (double precision float=w1058:T14)
        n523 = To Double Precision Float(number=w1077) -> (double precision float=w1081:T14)
        n524 = shared-variable "NI-cRIO9075-01756F19\\Shared Variables.lvlib\\Stage position"() -> (w991:dbl)  [unwired: 1 in, 1 out]
        "Stage position (mm):" <- w991
        n525 = Unbundle By Name(w1081) -> ("Channel 0"=w1046:dbl, "Channel 1"=w993:dbl, "Channel 2"=w992:dbl)
        n526 = Unbundle By Name(w1058) -> ("Channel 0"=w1035:dbl, "Channel 1"=w1051:dbl)
        n527 = Get Date/Time In Seconds() -> (seconds since 1Jan1904=w1055:timestamp)
        n528 = Multiply(x=1000.0, y=w1035) -> (x*y=w1034:dbl)
        n529 = To Double Precision Float(number=w1055) -> (double precision float=w1037:dbl)
        n530 = Build Array(w1034) -> (w1049:dbl[])
        n531 = Build Array(w1051) -> (w1050:dbl[])
        n532 = Build Array(w1046) -> (w1045:dbl[])
        n533 = Build Array(w993) -> (w1044:dbl[])
        n534 = Build Array(w992) -> (w1043:dbl[])
        n535 = Build Array(w991) -> (w990:dbl[])
        n536 = Build Array (concatenate)(w1054, w1037) -> (w1009:dbl[])
        n537 = Build Array (concatenate)(w1048, w1049) -> (w1013:dbl[])
        n538 = Build Array (concatenate)(w1047, w1050) -> (w1016:dbl[])
        n539 = Build Array (concatenate)(w1040, w1045) -> (w1019:dbl[])
        n540 = Build Array (concatenate)(w1039, w1044) -> (w1022:dbl[])
        n541 = Build Array (concatenate)(w1038, w1043) -> (w1025:dbl[])
        n542 = Build Array (concatenate)(w985, w990) -> (w989:dbl[])
        n543 = Divide(x=u32 40000000, y=w1029) -> (x/y=→"Control loop frequency (Hz)":dbl)
        n544 = call "Convert to Dynamic Data2"("Array"=w1016) -> ("Dynamic Data Type"=w1015:dynamicdata)  [unwired: 3 in]
        n545 = call "Convert to Dynamic Data6"("Array"=w1025) -> ("Dynamic Data Type"=w1024:dynamicdata)  [unwired: 3 in]
        n546 = call "Convert to Dynamic Data3"("Array"=w1019) -> ("Dynamic Data Type"=w1018:dynamicdata)  [unwired: 3 in]
        n547 = call "Convert to Dynamic Data4"("Array"=w1022) -> ("Dynamic Data Type"=w1021:dynamicdata)  [unwired: 3 in]
        n548 = call "Convert to Dynamic Data"("Array"=w1013) -> ("Dynamic Data Type"=w1012:dynamicdata)  [unwired: 3 in]
        n549 = call "Convert to Dynamic Data5"("Array"=w989) -> ("Dynamic Data Type"=w988:dynamicdata)  [unwired: 3 in]
        n550 = call "Filter"("Lower Cut-Off"=w986, "Signal"=w1015) -> ("Filtered Signal"=w1014:dynamicdata)  [unwired: 8 in, 1 out]
        n551 = call "Filter"("Lower Cut-Off"=w986, "Signal"=w1024) -> ("Filtered Signal"=w1023:dynamicdata)  [unwired: 8 in, 1 out]
        n552 = call "Filter"("Lower Cut-Off"=w986, "Signal"=w1018) -> ("Filtered Signal"=w1017:dynamicdata)  [unwired: 8 in, 1 out]
        n553 = call "Filter"("Lower Cut-Off"=w986, "Signal"=w1021) -> ("Filtered Signal"=w1020:dynamicdata)  [unwired: 8 in, 1 out]
        n554 = call "Filter"("Lower Cut-Off"=w986, "Signal"=w1012) -> ("Filtered Signal"=w1011:dynamicdata)  [unwired: 8 in, 1 out]
        n555 = call "Filter2"("Lower Cut-Off"=w986, "Signal"=w988) -> ("Filtered Signal"=w987:dynamicdata)  [unwired: 8 in, 1 out]
        n556 = call "Convert from Dynamic Data2"("Dynamic Data Type"=w1014) -> ("Array"=w1007:dbl[])  [unwired: 3 in]
        n557 = call "Convert from Dynamic Data6"("Dynamic Data Type"=w1023) -> ("Array"=w1004:dbl[])  [unwired: 3 in]
        n558 = call "Convert from Dynamic Data3"("Dynamic Data Type"=w1017) -> ("Array"=w1006:dbl[])  [unwired: 3 in]
        n559 = call "Convert from Dynamic Data4"("Dynamic Data Type"=w1020) -> ("Array"=w1005:dbl[])  [unwired: 3 in]
        n560 = call "Convert from Dynamic Data"("Dynamic Data Type"=w1011) -> ("Array"=w1008:dbl[])  [unwired: 3 in]
        n561 = call "Convert from Dynamic Data5"("Dynamic Data Type"=w987) -> ("Array"=w982:dbl[])  [unwired: 3 in]
        n562 = Array Size(array=w1009) -> (size(s)=w1056:i32)
        n563 = Greater?(x=w1056, y="Number of points") -> (0:w1057:bool)
        n564 = case shown="True" w1057 {
          tunnel: w1008 -> [w1111 w1126]
          tunnel: w1009 -> [w1112 w1128]
          tunnel: w1056 -> [_ w1129]
          tunnel: "Number of points" -> [_ w1115]
          tunnel: [w1112 w1127] -> w984
          tunnel: [w1111 w1125] -> w997
          tunnel: w1007 -> [w1110 w1123]
          tunnel: [w1110 w1124] -> w996
          tunnel: [w1107 w1122] -> w995
          tunnel: [w1109 w1121] -> w973
          tunnel: [w1108 w1120] -> w977
          tunnel: w1006 -> [w1107 w1119]
          tunnel: w1005 -> [w1109 w1118]
          tunnel: w1004 -> [w1108 w1117]
          tunnel: w982 -> [w1106 w1114]
          tunnel: [w1106 w1113] -> w981
          frame False {
          }
          frame True {
            n565 = Subtract(x=w1129, y=w1115) -> (x-y=w1116:i32)
            n566 = Array Subset(array=w1128, index=w1116, length=w1115) -> (w1127:dbl[])
            n567 = Array Subset(array=w1126, index=w1116, length=w1115) -> (w1125:dbl[])
            n568 = Array Subset(array=w1123, index=w1116, length=w1115) -> (w1124:dbl[])
            n569 = Array Subset(array=w1119, index=w1116, length=w1115) -> (w1122:dbl[])
            n570 = Array Subset(array=w1118, index=w1116, length=w1115) -> (w1121:dbl[])
            n571 = Array Subset(array=w1117, index=w1116, length=w1115) -> (w1120:dbl[])
            n572 = Array Subset(array=w1114, index=w1116, length=w1115) -> (w1113:dbl[])
          }
        }
        n573 = case shown="False" "Retain data" {
          tunnel: w1009 -> [_ w1105]
          tunnel: w1008 -> [_ w1104]
          tunnel: w1007 -> [_ w1103]
          tunnel: w1006 -> [_ w1102]
          tunnel: w1005 -> [_ w1101]
          tunnel: w1004 -> [_ w1100]
          tunnel: [w1093 w1105] -> w1003
          tunnel: [w1094 w1104] -> w1002
          tunnel: [w1095 w1103] -> w1001
          tunnel: [w1096 w1102] -> w1000
          tunnel: [w1097 w1101] -> w999
          tunnel: [w1098 w1100] -> w998
          tunnel: w984 -> [w1093 _]
          tunnel: w997 -> [w1094 _]
          tunnel: w996 -> [w1095 _]
          tunnel: w995 -> [w1096 _]
          tunnel: w973 -> [w1097 _]
          tunnel: w977 -> [w1098 _]
          tunnel: w982 -> [_ w1099]
          tunnel: [w1092 w1099] -> w980
          tunnel: w981 -> [w1092 _]
          frame False {
          }
          frame True {
          }
        }
        n574 = call <vilib>:"Std Deviation and Variance.vi"("X"=w973) -> ("mean"=→"F avg":dbl, "standard deviation"=→"F std":dbl)  [unwired: 1 in, 1 out]
        n575 = Array Size(array=w977) -> (size(s)=w978:i32)
        n576 = Bundle(w984, "Array"=w997) -> (w1053:cluster{dbl[], "Array":dbl[]})  [unwired: 1 in]
        n577 = Bundle(w984, "Array"=w996) -> (w1052:cluster{dbl[], "Array":dbl[]})  [unwired: 1 in]
        n578 = Bundle(w984, "Array"=w973) -> (w968:cluster{dbl[], "Array":dbl[]})  [unwired: 1 in]
        "Force (N)" <- w968
        n579 = Bundle(w984, "Array"=w995) -> (→"V*":cluster{dbl[], "Array":dbl[]})  [unwired: 1 in]
        n580 = Bundle(w984, "Array"=w977) -> (→"Roller position (mm)":cluster{dbl[], "Array":dbl[]})  [unwired: 1 in]
        n581 = Bundle(w984, "Array"=w981) -> (→"Stage position (mm)":cluster{dbl[], "Array":dbl[]})  [unwired: 1 in]
        n582 = Decrement(x=w978) -> (x-1=w979:i32)
        n583 = Build Array(w1053, w1052) -> (→"Inputs (mV or V)":cluster{dbl[], "Array":dbl[]}[])
        n584 = Index Array(array=w977, index=w979) -> (element=w976:dbl)
        n585 = Array Size(array=w973) -> (size(s)=w974:i32)
        n586 = Decrement(x=w974) -> (x-1=w975:i32)
        n587 = local read "Roller LED"() -> (w972:bool)
        n588 = Index Array(array=w973, index=w975) -> (element=w969:dbl)
        n589 = local read "Roller LED"() -> (w971:bool)
        n590 = local read "Test LED"() -> (w970:bool)
        n591 = case shown="True" w970 {
          tunnel: w969 -> [_ w1087]
          tunnel: w968 -> [_ w1086]
          frame False {
            n592 = local write "Measured contact force (N):"(0.0 ("Measured contact force (N):")) -> ()
            n593 = local write "Stage position (mm):"(0.0 ("Stage position (mm):")) -> ()
            n594 = local write "Force results (N)"(cluster{dbl[], dbl[]} {array[1000 elements], array[1000 elements]} ("Force results (N)")) -> ()
          }
          frame True {
            n595 = shared-variable "NI-cRIO9075-01756F19\\Shared Variables.lvlib\\Stage position"() -> (→"Stage position (mm):":dbl)  [unwired: 1 in, 1 out]
            "Measured contact force (N):" <- w1087
            "Force results (N)" <- w1086
          }
        }
        n596 = case shown="True" w972 {
          tunnel: w976 -> [_ w1091]
          frame False {
            n597 = local write "Position (mm):"(0.0 ("Position (mm):")) -> ()
          }
          frame True {
            "Position (mm):" <- w1091
          }
        }
        n598 = case shown="False" w971 {
          tunnel: w969 -> [_ w1089]
          frame False {
            n599 = local write "Force (N):"(0.0 ("Force (N):")) -> ()
          }
          frame True {
            "Force (N):" <- w1089
          }
        }
        n600 = call "UI Error Handler - Monitoring.vi"("error in (no error)"=w958, "Message Queue"=w1063) -> ()  [unwired: 9 in, 1 out]
      }
    }
    n601 = global read "Global - All UI Loop Stop.vi" "All UI Loop Stop"() -> (w911:bool)
  }
  n602 = Unregister For Events(event registration refnum=w14, error in=w22) -> (error out=w15:errorcluster)
  n603 = Merge Errors(w15, w23) -> (w21:errorcluster)
  n604 = call "Destroy User Event - Stop.vi"("error in (no error)"=w21, "User Event - Stop"=w19) -> ("error out"=w12:errorcluster)  [unwired: 9 in]
  n605 = call <vilib>:"Simple Error Handler.vi"("error in (no error)"=w12) -> ()  [unwired: 4 in, 5 out]
  "Max position (mm):" <- 151.49760546875
  "Max speed (mm/s):" <- 21.0 ("Max speed (mm/s):")
